vi "Match_Gauge Block.vi"(4 "Data in":string[][](array[string]), 5 "Calibration Default":string[][](array[string]), 6 "세부분류코드":string, 7 "Cal STD":string[][](array[string]), 8 "에러 입력":errorcluster caption="에러 입력(에러 없음)", 11 "Func_ext in":string) -> (0 "에러 출력":errorcluster, 1 "Data Out 2":string[](array[string]), 2 "Data Out":string[][](array[string]), 3 "CalSTD":string[][](array[string]))   [LabVIEW 2020]
uses:
  Controls/Cmd_File path.ctl
  Controls/Cmd_File Type.ctl
  Controls/Cmd_Var Data IO.ctl
  <vilib>/Utility/file.llb/Read Delimited Spreadsheet (string).vi
  Public/Polymorph/Data Class_2D Str.vi
  Public/Polymorph/Array Dedup_2D Str.vi
  Variables/Global_Cal Info.vi
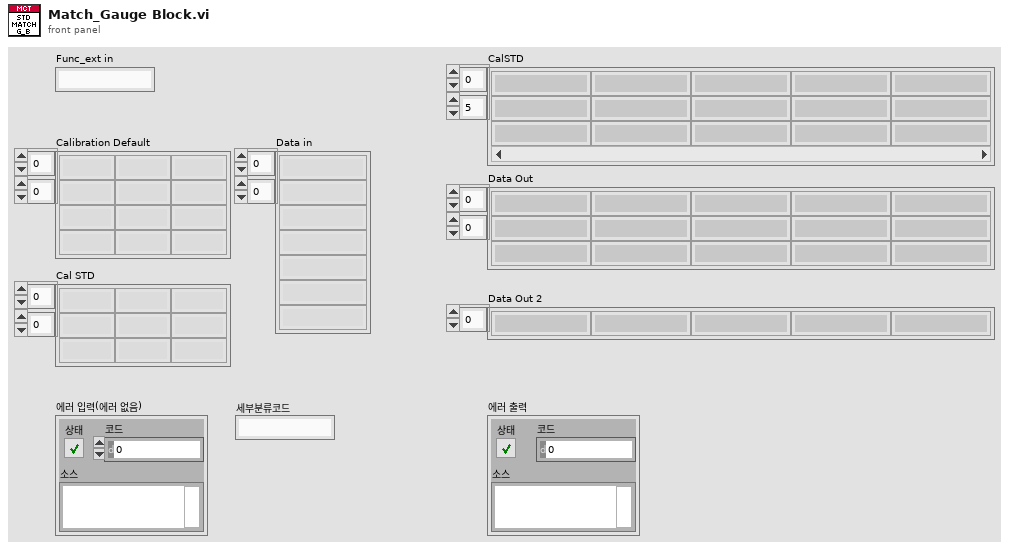
[diagram p1: front panel]
types:
  T1 = typedef "Cmd_File Type.ctl" = enum16{"엑셀", "엑셀(2003)", "텍스트", "설정", "2진", "VI", "CSV", "LOG", "폴더"}
  T2 = typedef "Cmd_File path.ctl" = enum16{"에러로그", "데이터파일경로", "성적서원본", "지난성적서", "Data Files", "경로생성", "Updater", "Template", "설정파일경로", "FTP Upload", "Update 경로", "어플리케이션"}
  T3 = typedef "Cmd_Var Data IO.ctl" = enum16{"Condition", "Condition Default", "Condition_Temp", "Resolution", "Resolution Default", "Resolution Old", "Spec", "Spec Default", "Spec Old", "Spec Temp", "Result", "Result2", "Result3", "Result_Temp", "Result_ADJ", "Result_ADJ2", "STD1", "STD2", "STD3", "STD4", "STD5", "STD Temp", "CMC", "CMC Default"}
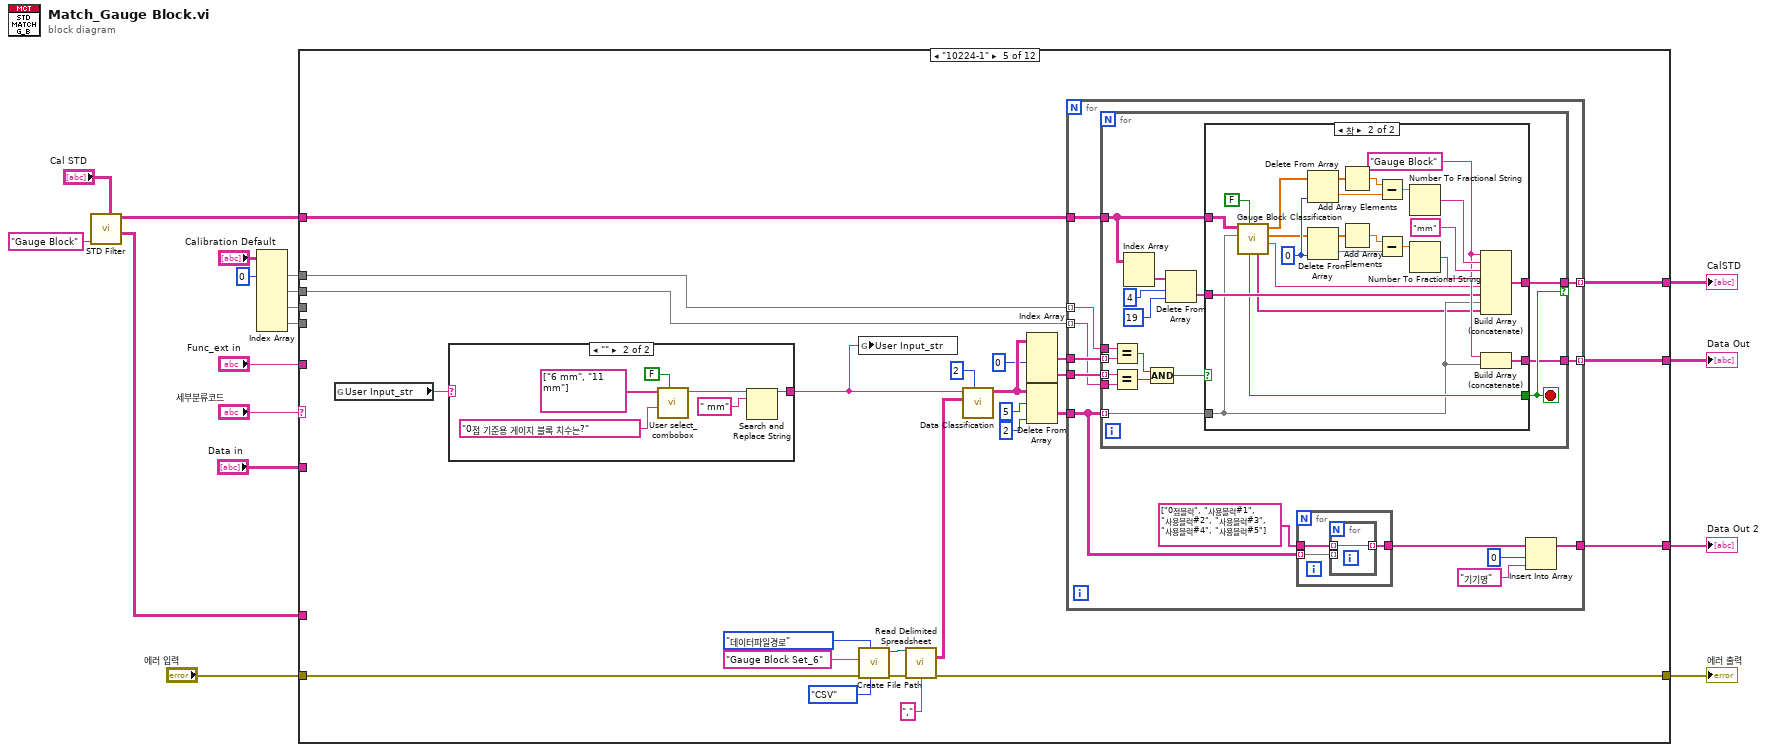
[diagram p0: block diagram]
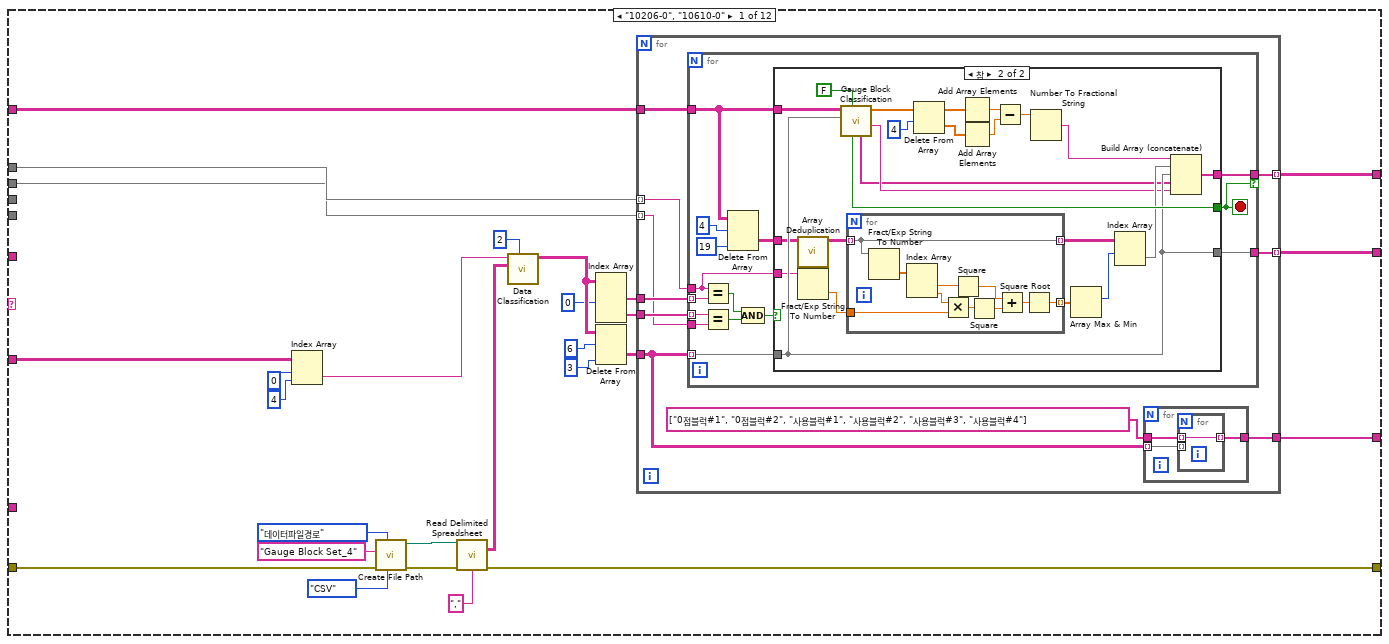
[diagram p2: hidden frame]
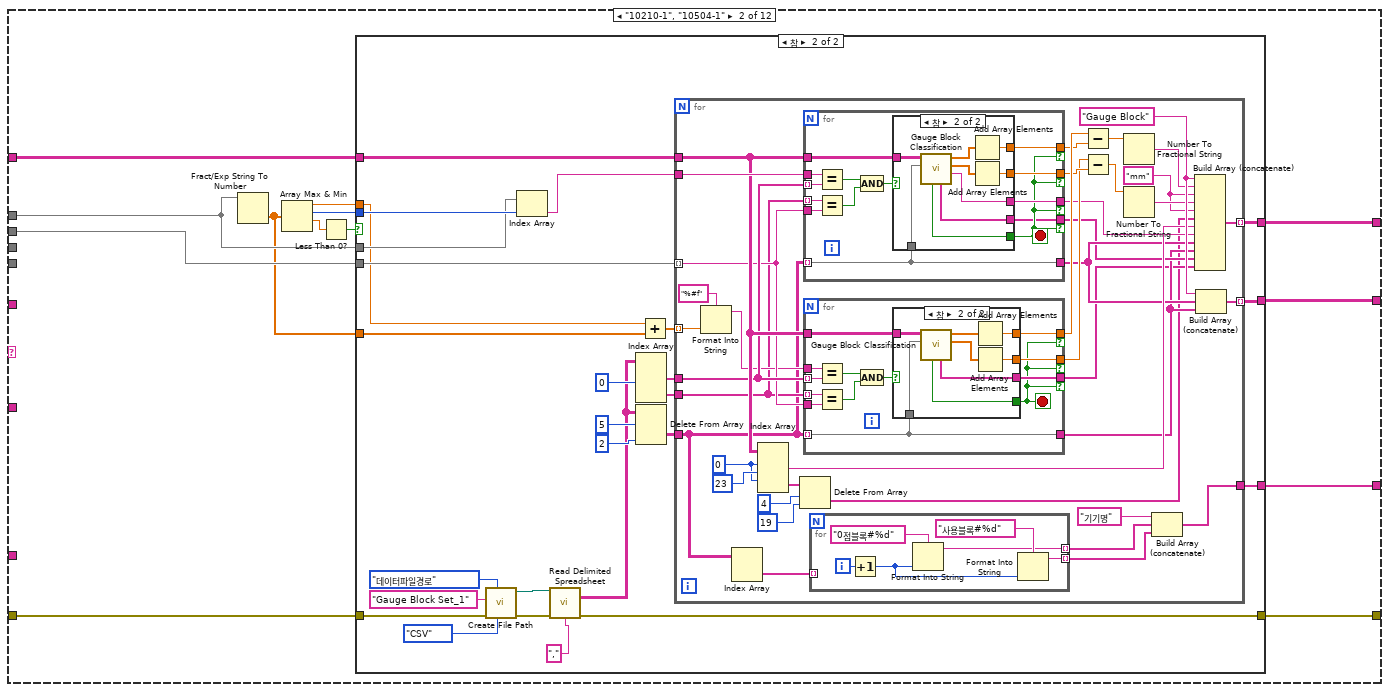
[diagram p4: hidden frame]
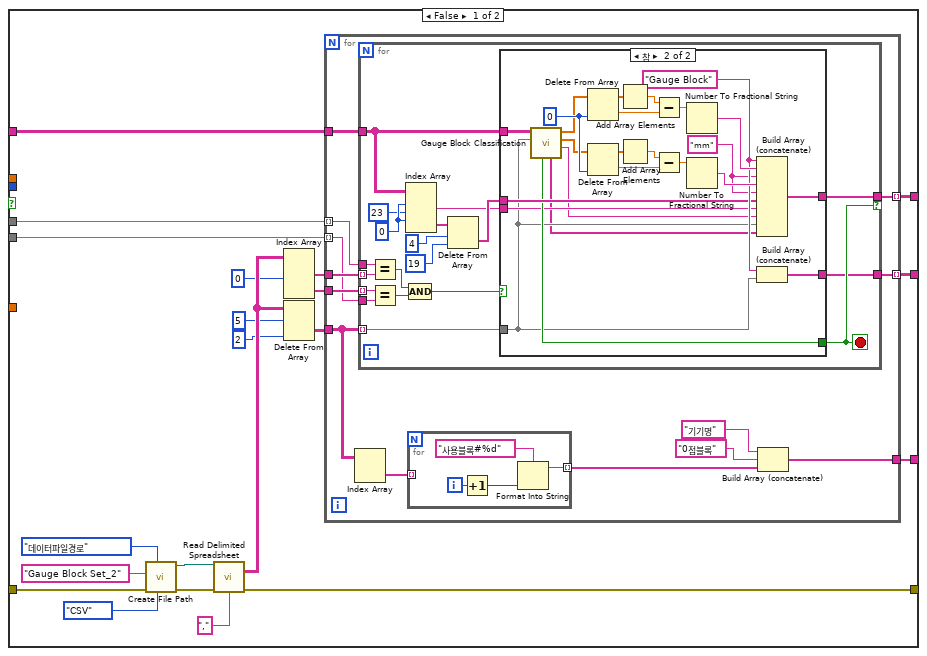
[diagram p5: hidden frame]
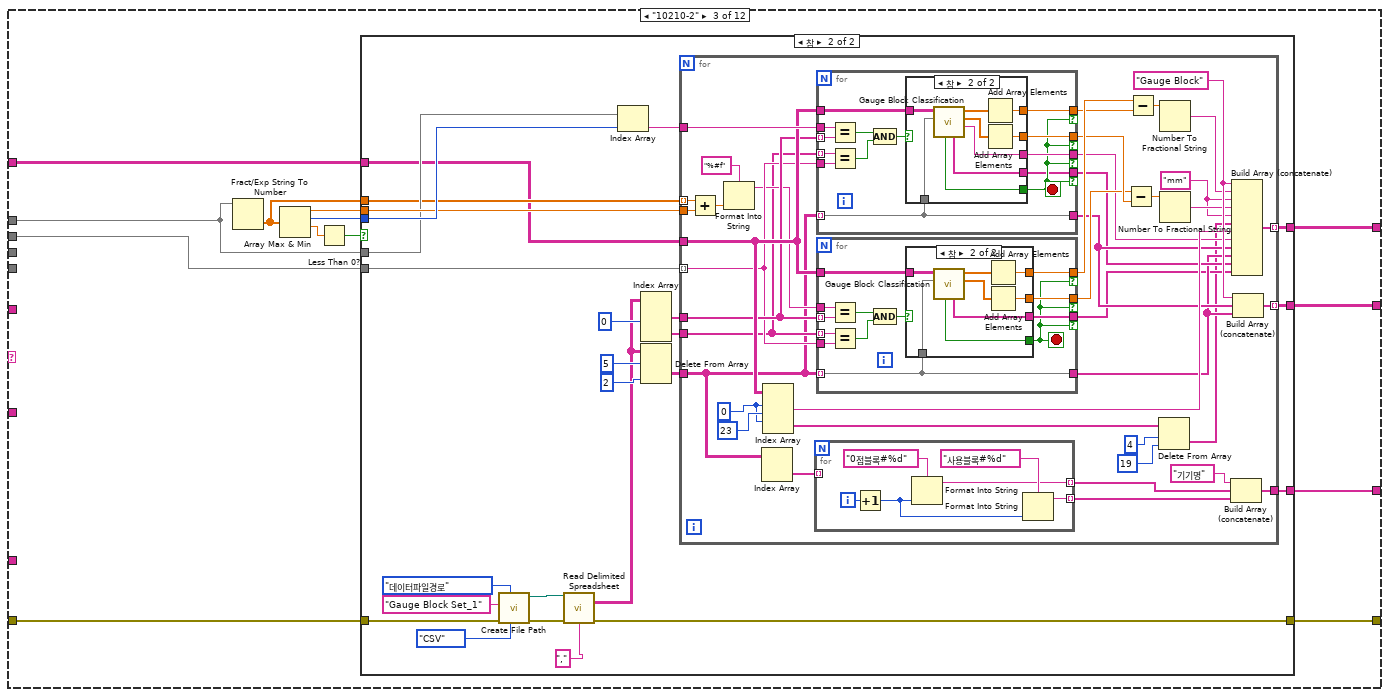
[diagram p9: hidden frame]
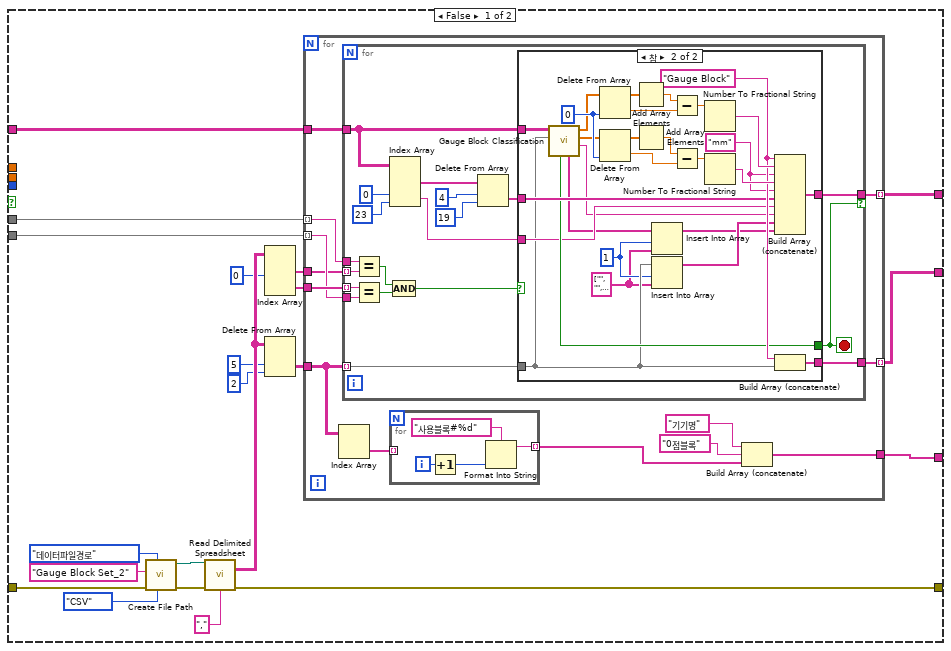
[diagram p10: hidden frame]
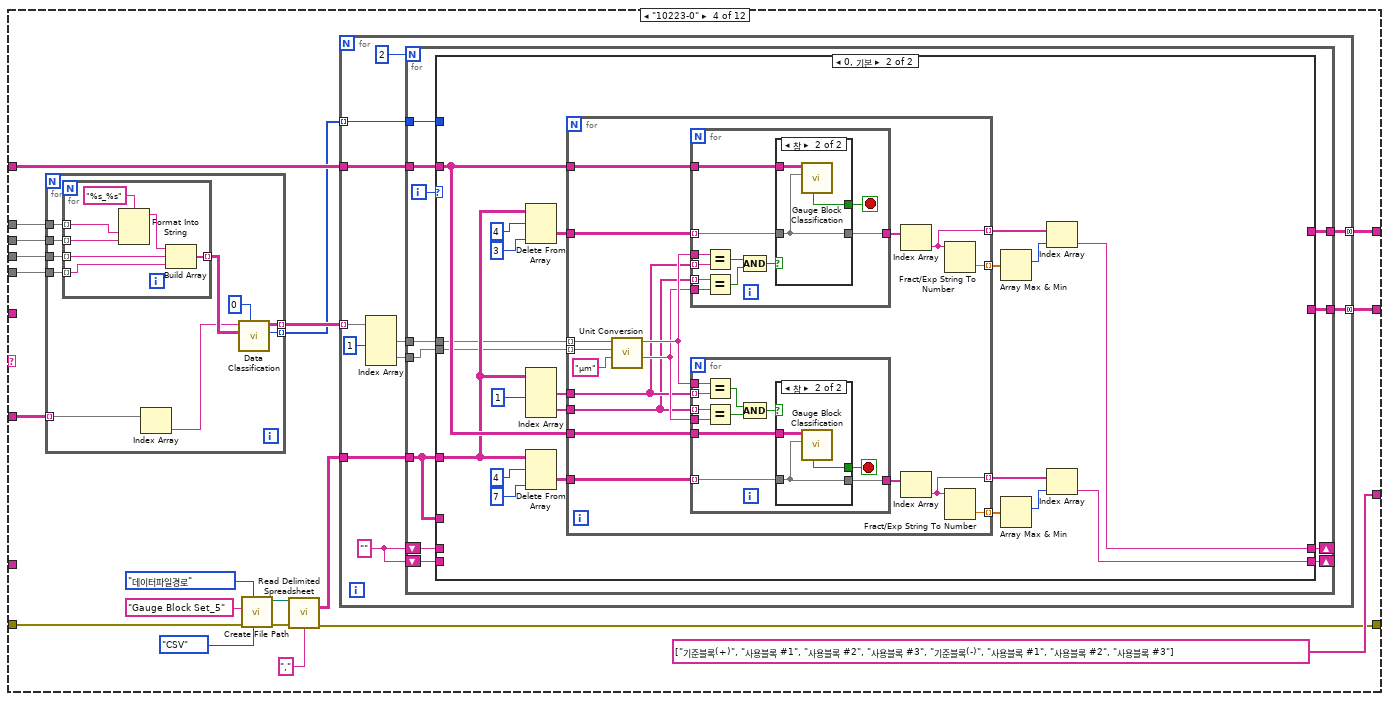
[diagram p14: hidden frame]
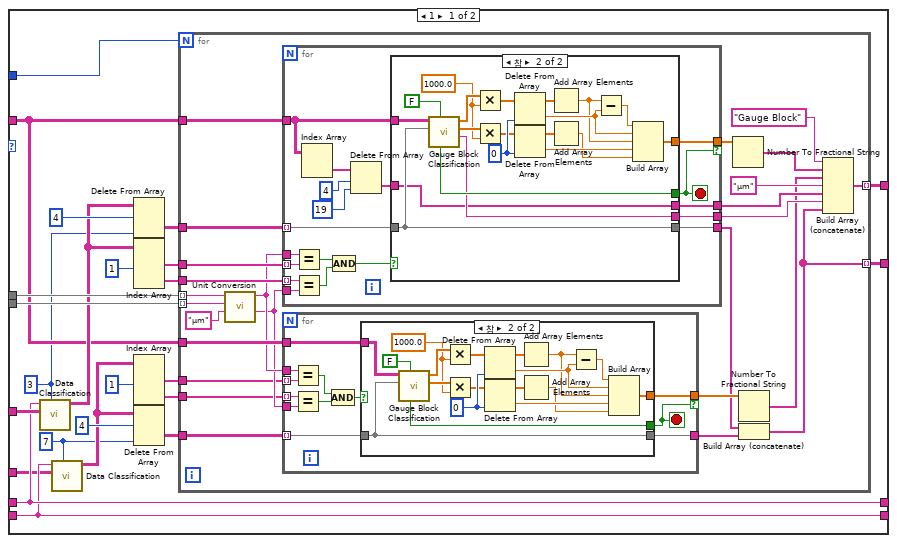
[diagram p15: hidden frame]
diagram:
  n1 = call "STD Filter.vi"("Cal STD in"="Cal STD", "문자열(option, STD)"="Gauge Block" ("검색 문자열")) -> ("Cal STD out"=w6:string[][], "DATA 출력"=w7:string[][])  [unwired: 5 in, 3 out]
  n2 = Index Array(array="Calibration Default", index (col) #1=0 ("비활성화된 인덱스 (열)")) -> (element #1=w10:string[], element #2=w9:string[], element #3=w2:string[], element #4=w1:string[])  [unwired: 7 in]
  n3 = case shown="\"10224-1\"" "세부분류코드" {
    tunnel: w10 -> [w28 w111 w326 w532 w782 w882 _ w1052 w1142 w1266 w1347 w1436]
    tunnel: w9 -> [w27 w112 w328 w531 w781 w881 w951 w1051 w1141 w1265 w1346 w1435]
    tunnel: w6 -> [_ _ _ _ _ w866 w957 _ _ w1250 w1331 w1420]
    tunnel: [w21 w120 w317 w548 w780 w880 w971 w1050 w1140 w1264 w1345 w1434] -> w13
    tunnel: [w20 w119 w318 w547 w779 w879 w970 w1049 w1139 w1263 w1344 w1433] -> w14
    tunnel: [w22 w116 w320 w535 w773 w861 w952 w1039 w1129 w1245 w1326 w1415] -> w16
    tunnel: "에러 입력" -> [w24 w118 w321 w537 w772 w864 w955 w1048 w1138 w1248 w1329 w1418]
    tunnel: [w19 w117 w319 string[] ["기준블록(+)", "사용블록 #1", "사용블록 #2", "사용블록 #3", "기준블록(-)", "사용블록 #1", "사용블록 #2", "사용블록 #3"] w778 w874 w965 w1043 w1133 w1258 w1339 w1428] -> w15
    tunnel: "Func_ext in" -> [_ _ _ _ _ w868 w959 _ _ w1252 w1333 w1422]
    tunnel: w7 -> [w26 w108 w316 w545 w775 w863 w954 w1041 w1131 w1247 w1328 w1417]
    tunnel: "Data in" -> [w25 _ _ w533 _ _ _ _ _ _ _ _]
    tunnel: w2 -> [_ _ _ w530 _ _ w950 _ _ _ _ _]
    tunnel: w1 -> [_ _ _ w529 _ _ _ _ _ _ _ _]
    frame "10206-0", "10610-0" {
      n4 = Index Array(array=w25, index (row)=0 ("인덱스 (행)"), index (col)=4 ("비활성화된 인덱스 (열)")) -> (element=w44:string)
      n5 = call "Create File Path.vi"("파일타입"=Cmd_File_Type."CSV", "항목"=Cmd_File_path."데이터파일경로", "에러 입력"=w24, "문자열 in"="Gauge Block Set_4" ("delimiter (\\t)")) -> ("error out"=w23:errorcluster, "파일경로"=w38:path)  [unwired: 4 in, 2 out]
      n6 = call-poly <vilib>:"Read Delimited Spreadsheet.vi"("file path (dialog if empty)"=w38, "error in (no error)"=w23, "delimiter (\\t)"="," ("delimiter (\\t)")) -> ("all rows"=w45:string[][], "error out"=w22:errorcluster)  [unwired: 7 in, 4 out]
      n7 = call-poly "Data Classification.vi"("인덱스"=2, "DATA 입력"=w45, "검색 문자열"=w44) -> ("DATA 출력"=w41:string[][])  [unwired: 4 in, 4 out]
      n8 = Index Array(array=w41, index (col) #1=0 ("비활성화된 인덱스 (열)")) -> (element #1=w30:string[], element #2=w29:string[])  [unwired: 3 in]
      n9 = Delete From Array(array=w41, length=6 ("길이"), index (col)=3 ("비활성화된 인덱스 (열)")) -> (deleted portion=w32:string[][])  [unwired: 1 in, 1 out]
      n10 = for {
        tunnel: w32 -> [w47]
        tunnel: w26 -> [w55]
        tunnel: w28 -> [w54] mode=indexing
        tunnel: w30 -> [w53]
        tunnel: w29 -> [w52]
        tunnel: w27 -> [w51] mode=indexing
        tunnel: [w50] -> w21 mode=indexing
        tunnel: [w49] -> w20 mode=indexing
        tunnel: [w46] -> w19
        n11 = for {
          tunnel: w54 -> [w56]
          tunnel: w51 -> [w70]
          tunnel: w47 -> [w67] mode=indexing
          tunnel: w55 -> [w60]
          tunnel: [w65] -> w50 if=w64
          tunnel: [w63] -> w49
          tunnel: w53 -> [w62] mode=indexing
          tunnel: w52 -> [w61] mode=indexing
          stop <- w64 stop-if-true
          n12 = Equal?(x=w56, y=w62) -> (x = y?=w68:bool)
          n13 = Equal?(x=w61, y=w70) -> (x = y?=w69:bool)
          n14 = Delete From Array(array=w60, length=4 ("길이"), index (col)=19 ("비활성화된 인덱스 (열)")) -> (deleted portion=w57:string[][])  [unwired: 1 in, 1 out]
          n15 = Compound Arithmetic op=AND(w68, w69) -> (w66:bool)
          n16 = case shown="참" w66 {
            tunnel: w67 -> [_ w87]
            tunnel: [_ w91] -> w64
            tunnel: w60 -> [_ w93]
            tunnel: [_ w92] -> w65
            tunnel: [_ w87] -> w63
            tunnel: w57 -> [_ w83]
            tunnel: w56 -> [_ w82]
            frame False {
            }
            frame True {
              n17 = call-poly "Array Deduplication.vi"("배열 in"=w83) -> ("배열 out"=w80:string[][])  [unwired: 9 in, 1 out]
              n18 = Fract/Exp String To Number(string=w82) -> (number=w81:dbl)  [unwired: 3 in, 1 out]
              n19 = call "Gauge Block Classification.vi"("블록삭제?(T)"=FALSE, "블록리스트"=w87, "게이지 블록 교정data"=w93) -> ("열팽창계수"=w73:string, "블록치수"=w88:dbl[], "교정값(문자)"=w72:string[], "stop?"=w91:bool)  [unwired: 3 in, 2 out]
              n20 = for {
                tunnel: w80 -> [w94] mode=indexing
                tunnel: w81 -> [w102]
                tunnel: [w95] -> w79 mode=indexing
                tunnel: [w94] -> w78 mode=indexing
                n21 = Fract/Exp String To Number(string=w94) -> (number=w103:dbl[])  [unwired: 3 in, 1 out]
                n22 = Index Array(array=w103) -> (element #1=w100:dbl, element #2=w101:dbl)  [unwired: 2 in]
                n23 = Multiply(x=w101, y=w102) -> (x*y=w99:dbl)
                n24 = Square(x=w100) -> (x^2=w98:dbl)
                n25 = Square(x=w99) -> (x^2=w97:dbl)
                n26 = Add(x=w98, y=w97) -> (x+y=w96:dbl)
                n27 = Square Root(x=w96) -> (sqrt(x)=w95:dbl)
              }
              n28 = Delete From Array(array=w88, length=4 ("길이")) -> (deleted portion=w90:dbl[], array with subset deleted=w75:dbl[])  [unwired: 1 in]
              n29 = Add Array Elements(numeric array=w75) -> (sum=w74:dbl)
              n30 = Add Array Elements(numeric array=w90) -> (sum=w84:dbl)
              n31 = Subtract(x=w74, y=w84) -> (x-y=w85:dbl)
              n32 = Number To Fractional String(number=w85) -> (F-format string=w89:string)  [unwired: 3 in]
              n33 = Array Max & Min(array=w79) -> (max index (indices)=w77:i32)  [unwired: 3 out]
              n34 = Index Array(array=w78, index (row)=w77) -> (element=w76:string[])  [unwired: 1 in]
              n35 = Build Array (concatenate)(w89, w76, w87, w72, w73) -> (w92:string[])
            }
          }
        }
        n36 = for {
          tunnel: w47 -> [w105] mode=indexing
          tunnel: string[] ["0점블럭#1", "0점블럭#2", "사용블럭#1", "사용블럭#2", "사용블럭#3", "사용블럭#4"] -> [w106]
          tunnel: [w104] -> w46
          n37 = for {
            tunnel: w106 -> [w107] mode=indexing
            tunnel: w105 -> [_] mode=indexing
            tunnel: [w107] -> w104 mode=indexing
          }
        }
      }
    }
    frame "10210-1", "10504-1" {
      n38 = Fract/Exp String To Number(string=w111) -> (number=w110:dbl[])  [unwired: 3 in, 1 out]
      n39 = Array Max & Min(array=w110) -> (max value=w113:dbl, max index (indices)=w114:i32, min value=w115:dbl)  [unwired: 1 out]
      n40 = Less Than 0?(x=w115) -> (x < 0?=w109:bool)
      n41 = case shown="참" w109 {
        tunnel: w108 -> [w129 w227]
        tunnel: [w125 w219] -> w120
        tunnel: [w124 w218] -> w119
        tunnel: w118 -> [w126 w217]
        tunnel: [w123 w212] -> w117
        tunnel: [w121 w202] -> w116
        tunnel: w114 -> [_ w209]
        tunnel: w113 -> [_ w206]
        tunnel: w112 -> [w128 w208]
        tunnel: w111 -> [w127 w207]
        tunnel: w110 -> [_ w205]
        frame False {
          n42 = call "Create File Path.vi"("파일타입"=Cmd_File_Type."CSV", "항목"=Cmd_File_path."데이터파일경로", "에러 입력"=w126, "문자열 in"="Gauge Block Set_2" ("delimiter (\\t)")) -> ("error out"=w122:errorcluster, "파일경로"=w140:path)  [unwired: 4 in, 2 out]
          n43 = call-poly <vilib>:"Read Delimited Spreadsheet.vi"("file path (dialog if empty)"=w140, "error in (no error)"=w122, "delimiter (\\t)"="," ("delimiter (\\t)")) -> ("all rows"=w141:string[][], "error out"=w121:errorcluster)  [unwired: 7 in, 4 out]
          n44 = Index Array(array=w141, index (col) #1=0 ("비활성화된 인덱스 (열)")) -> (element #1=w138:string[], element #2=w137:string[])  [unwired: 3 in]
          n45 = Delete From Array(array=w141, length=5 ("길이"), index (col)=2 ("비활성화된 인덱스 (열)")) -> (deleted portion=w139:string[][])  [unwired: 1 in, 1 out]
          n46 = for {
            tunnel: w139 -> [w144]
            tunnel: w129 -> [w154]
            tunnel: w127 -> [w153] mode=indexing
            tunnel: w138 -> [w152]
            tunnel: w137 -> [w151]
            tunnel: w128 -> [w150] mode=indexing
            tunnel: [w149] -> w125 mode=indexing
            tunnel: [w148] -> w124 mode=indexing
            tunnel: [w145] -> w123
            n47 = Index Array(array=w144) -> (element=w143:string[])  [unwired: 2 in]
            n48 = for {
              tunnel: w153 -> [w177]
              tunnel: w150 -> [w176]
              tunnel: w144 -> [w173] mode=indexing
              tunnel: w154 -> [w163]
              tunnel: [w171] -> w149 if=w170
              tunnel: [w169] -> w148
              tunnel: w152 -> [w168] mode=indexing
              tunnel: w151 -> [w167] mode=indexing
              stop <- w170 stop-if-true
              w161 = 0 ("인덱스 (행)")
              n49 = Equal?(x=w177, y=w168) -> (x = y?=w174:bool)
              n50 = Equal?(x=w167, y=w176) -> (x = y?=w175:bool)
              n51 = Index Array(array=w163, index (row) #1=w161, index (col) #1=23 ("비활성화된 인덱스 (열)"), index (row) #2=w161) -> (element #1=w159:string, element #2=w165:string[])  [unwired: 1 in]
              n52 = Compound Arithmetic op=AND(w174, w175) -> (w172:bool)
              n53 = Delete From Array(array=w165, length=4 ("길이"), index=19 ("비활성화된 인덱스 (열)")) -> (deleted portion=w162:string[])  [unwired: 1 out]
              n54 = case shown="참" w172 {
                tunnel: w173 -> [_ w179]
                tunnel: [_ w184] -> w170
                tunnel: w163 -> [_ w183]
                tunnel: [_ w201] -> w171
                tunnel: [_ w197] -> w169
                tunnel: w162 -> [_ w187]
                tunnel: w159 -> [_ w182]
                frame False {
                }
                frame True {
                  w190 = 0 ("인덱스")
                  w180 = "mm" ("환산단위")
                  w198 = "Gauge Block" ("검색 문자열")
                  n55 = call "Gauge Block Classification.vi"("블록리스트"=w179, "게이지 블록 교정data"=w183) -> ("열팽창계수"=w181:string, "교정값(값)"=w185:dbl[], "블록치수"=w186:dbl[], "교정값(문자)"=w178:string[], "stop?"=w184:bool)  [unwired: 4 in, 1 out]
                  n56 = Delete From Array(array=w186, index=w190) -> (deleted portion=w196:dbl, array with subset deleted=w192:dbl[])  [unwired: 1 in]
                  n57 = Delete From Array(array=w185, index=w190) -> (deleted portion=w194:dbl, array with subset deleted=w191:dbl[])  [unwired: 1 in]
                  n58 = Add Array Elements(numeric array=w192) -> (sum=w195:dbl)
                  n59 = Add Array Elements(numeric array=w191) -> (sum=w193:dbl)
                  n60 = Subtract(x=w195, y=w196) -> (x-y=w189:dbl)
                  n61 = Subtract(x=w193, y=w194) -> (x-y=w188:dbl)
                  n62 = Number To Fractional String(number=w189) -> (F-format string=w199:string)  [unwired: 3 in]
                  n63 = Number To Fractional String(number=w188) -> (F-format string=w200:string)  [unwired: 3 in]
                  n64 = Build Array (concatenate)(w198, w199, w180, w200, w180, w187, w182, w181, w179, w178) -> (w201:string[])
                  n65 = Build Array (concatenate)(w198, w179) -> (w197:string[])
                }
              }
            }
            n66 = for {
              tunnel: [w156] -> w147 mode=indexing
              tunnel: w143 -> [_] mode=indexing
              i -> [w157]
              n67 = Increment(x=w157) -> (x+1=w155:i32)
              n68 = Format Into String(format string="사용블록#%d" ("포맷 문자열"), w155) -> (resulting string=w156:string)  [unwired: 2 in, 1 out]
            }
            n69 = Build Array (concatenate)("기기명", "0점블록" ("포맷 문자열"), w147) -> (w145:string[])
          }
        }
        frame True {
          n70 = call "Create File Path.vi"("파일타입"=Cmd_File_Type."CSV", "항목"=Cmd_File_path."데이터파일경로", "에러 입력"=w217, "문자열 in"="Gauge Block Set_1" ("delimiter (\\t)")) -> ("error out"=w203:errorcluster, "파일경로"=w214:path)  [unwired: 4 in, 2 out]
          n71 = Index Array(array=w207, index=w209) -> (element=w210:string)
          n72 = call-poly <vilib>:"Read Delimited Spreadsheet.vi"("file path (dialog if empty)"=w214, "error in (no error)"=w203, "delimiter (\\t)"="," ("delimiter (\\t)")) -> ("all rows"=w211:string[][], "error out"=w202:errorcluster)  [unwired: 7 in, 4 out]
          n73 = Index Array(array=w211, index (col) #1=0 ("비활성화된 인덱스 (열)")) -> (element #1=w225:string[], element #2=w226:string[])  [unwired: 3 in]
          n74 = Delete From Array(array=w211, length=5 ("길이"), index (col)=2 ("비활성화된 인덱스 (열)")) -> (deleted portion=w223:string[][])  [unwired: 1 in, 1 out]
          n75 = Add(x=w206, y=w205) -> (x+y=w204:dbl[])
          n76 = for {
            tunnel: w223 -> [w232]
            tunnel: w227 -> [w262]
            tunnel: w225 -> [w261]
            tunnel: w226 -> [w239]
            tunnel: w208 -> [w260] mode=indexing
            tunnel: [w265] -> w219 mode=indexing
            tunnel: [w264] -> w218 mode=indexing
            tunnel: [w235] -> w212
            tunnel: w210 -> [w263]
            tunnel: w204 -> [w229] mode=indexing
            w243 = 0 ("인덱스 (행)")
            w228 = "mm" ("환산단위")
            w257 = "Gauge Block" ("검색 문자열")
            n77 = Format Into String(format string="%#f" ("포맷 문자열"), w229) -> (resulting string=w258:string)  [unwired: 2 in, 1 out]
            n78 = Index Array(array=w232) -> (element=w231:string[])  [unwired: 2 in]
            n79 = Index Array(array=w262, index (row) #1=w243, index (col) #1=23 ("비활성화된 인덱스 (열)"), index (row) #2=w243) -> (element #1=w247:string, element #2=w242:string[])  [unwired: 1 in]
            n80 = Delete From Array(array=w242, length=4 ("길이"), index=19 ("비활성화된 인덱스 (열)")) -> (deleted portion=w230:string[])  [unwired: 1 out]
            n81 = for {
              tunnel: w263 -> [w306]
              tunnel: w260 -> [w305]
              tunnel: w232 -> [w296] mode=indexing
              tunnel: w262 -> [w299]
              tunnel: [w293] -> w244 if=w294
              tunnel: [w296] -> w246
              tunnel: w261 -> [w301] mode=indexing
              tunnel: w239 -> [w300] mode=indexing
              tunnel: [w298] -> w252 if=w294
              tunnel: [w297] -> w253 if=w294
              tunnel: [w295] -> w245 if=w294
              stop <- w294 stop-if-true
              n82 = Equal?(x=w306, y=w301) -> (x = y?=w303:bool)
              n83 = Equal?(x=w300, y=w305) -> (x = y?=w304:bool)
              n84 = Compound Arithmetic op=AND(w303, w304) -> (w302:bool)
              n85 = case shown="참" w302 {
                tunnel: w296 -> [_ w312]
                tunnel: [_ w315] -> w294
                tunnel: w299 -> [_ w313]
                tunnel: [_ w311] -> w298
                tunnel: [_ w309] -> w297
                tunnel: [_ w308] -> w295
                tunnel: [_ w307] -> w293
                frame False {
                }
                frame True {
                  n86 = call "Gauge Block Classification.vi"("블록리스트"=w312, "게이지 블록 교정data"=w313) -> ("열팽창계수"=w308:string, "교정값(값)"=w314:dbl[], "블록치수"=w310:dbl[], "교정값(문자)"=w307:string[], "stop?"=w315:bool)  [unwired: 4 in, 1 out]
                  n87 = Add Array Elements(numeric array=w310) -> (sum=w309:dbl)
                  n88 = Add Array Elements(numeric array=w314) -> (sum=w311:dbl)
                }
              }
            }
            n89 = for {
              tunnel: w258 -> [w284]
              tunnel: w260 -> [w283]
              tunnel: w232 -> [w272] mode=indexing
              tunnel: w262 -> [w276]
              tunnel: [w279] -> w233 if=w273
              tunnel: [w272] -> w234
              tunnel: w261 -> [w278] mode=indexing
              tunnel: w239 -> [w277] mode=indexing
              tunnel: [w275] -> w256 if=w273
              tunnel: [w274] -> w251 if=w273
              stop <- w273 stop-if-true
              n90 = Equal?(x=w284, y=w278) -> (x = y?=w281:bool)
              n91 = Equal?(x=w277, y=w283) -> (x = y?=w282:bool)
              n92 = Compound Arithmetic op=AND(w281, w282) -> (w280:bool)
              n93 = case shown="참" w280 {
                tunnel: w272 -> [_ w288]
                tunnel: [_ w292] -> w273
                tunnel: w276 -> [_ w289]
                tunnel: [_ w285] -> w279
                tunnel: [_ w287] -> w275
                tunnel: [_ w286] -> w274
                frame False {
                }
                frame True {
                  n94 = call "Gauge Block Classification.vi"("블록리스트"=w288, "게이지 블록 교정data"=w289) -> ("교정값(값)"=w290:dbl[], "블록치수"=w291:dbl[], "교정값(문자)"=w285:string[], "stop?"=w292:bool)  [unwired: 4 in, 2 out]
                  n95 = Add Array Elements(numeric array=w291) -> (sum=w287:dbl)
                  n96 = Add Array Elements(numeric array=w290) -> (sum=w286:dbl)
                }
              }
            }
            n97 = for {
              tunnel: [w268] -> w238 mode=indexing
              tunnel: [w267] -> w237 mode=indexing
              tunnel: w231 -> [_] mode=indexing
              i -> [w269]
              n98 = Increment(x=w269) -> (x+1=w266:i32)
              n99 = Format Into String(format string="0점블록#%d" ("포맷 문자열"), w266) -> (resulting string=w268:string)  [unwired: 2 in, 1 out]
              n100 = Format Into String(format string="사용블록#%d" ("포맷 문자열"), w266) -> (resulting string=w267:string)  [unwired: 2 in, 1 out]
            }
            n101 = Subtract(x=w256, y=w253) -> (x-y=w255:dbl)
            n102 = Subtract(x=w251, y=w252) -> (x-y=w250:dbl)
            n103 = Number To Fractional String(number=w255) -> (F-format string=w254:string)  [unwired: 3 in]
            n104 = Number To Fractional String(number=w250) -> (F-format string=w249:string)  [unwired: 3 in]
            n105 = Build Array (concatenate)("기기명", w238, w237) -> (w235:string[])
            n106 = Build Array (concatenate)(w257, w254, w228, w249, w228, w230, w247, w245, w246, w234, w244, w233) -> (w265:string[])
            n107 = Build Array (concatenate)(w257, w246, w234) -> (w264:string[])
          }
        }
      }
    }
    frame "10210-2" {
      n108 = Fract/Exp String To Number(string=w326) -> (number=w322:dbl[])  [unwired: 3 in, 1 out]
      n109 = Array Max & Min(array=w322) -> (max value=w325:dbl, max index (indices)=w324:i32, min value=w327:dbl)  [unwired: 1 out]
      n110 = Less Than 0?(x=w327) -> (x < 0?=w323:bool)
      n111 = case shown="참" w323 {
        tunnel: [w336 w431] -> w317
        tunnel: [w335 w430] -> w318
        tunnel: w321 -> [w337 w429]
        tunnel: [w334 w424] -> w319
        tunnel: [w329 w414] -> w320
        tunnel: w324 -> [_ w421]
        tunnel: w325 -> [_ w420]
        tunnel: w328 -> [w339 w419]
        tunnel: w326 -> [w338 w418]
        tunnel: w322 -> [_ w417]
        tunnel: w316 -> [w331 w416]
        frame False {
          n112 = call "Create File Path.vi"("파일타입"=Cmd_File_Type."CSV", "항목"=Cmd_File_path."데이터파일경로", "에러 입력"=w337, "문자열 in"="Gauge Block Set_2" ("delimiter (\\t)")) -> ("error out"=w330:errorcluster, "파일경로"=w348:path)  [unwired: 4 in, 2 out]
          n113 = call-poly <vilib>:"Read Delimited Spreadsheet.vi"("file path (dialog if empty)"=w348, "error in (no error)"=w330, "delimiter (\\t)"="," ("delimiter (\\t)")) -> ("all rows"=w349:string[][], "error out"=w329:errorcluster)  [unwired: 7 in, 4 out]
          n114 = Index Array(array=w349, index (col) #1=0 ("비활성화된 인덱스 (열)")) -> (element #1=w333:string[], element #2=w332:string[])  [unwired: 3 in]
          n115 = Delete From Array(array=w349, length=5 ("길이"), index (col)=2 ("비활성화된 인덱스 (열)")) -> (deleted portion=w347:string[][])  [unwired: 1 in, 1 out]
          n116 = for {
            tunnel: w347 -> [w354]
            tunnel: w331 -> [w362]
            tunnel: w338 -> [w350] mode=indexing
            tunnel: w333 -> [w351]
            tunnel: w332 -> [w361]
            tunnel: w339 -> [w360] mode=indexing
            tunnel: [w359] -> w336 mode=indexing
            tunnel: [w358] -> w335 mode=indexing
            tunnel: [w355] -> w334
            n117 = Index Array(array=w354) -> (element=w353:string[])  [unwired: 2 in]
            n118 = for {
              tunnel: w350 -> [w385]
              tunnel: w360 -> [w384]
              tunnel: w354 -> [w382] mode=indexing
              tunnel: w362 -> [w373]
              tunnel: [w380] -> w359 if=w368
              tunnel: [w379] -> w358
              tunnel: w351 -> [w378] mode=indexing
              tunnel: w361 -> [w377] mode=indexing
              stop <- w368 stop-if-true
              n119 = Equal?(x=w385, y=w378) -> (x = y?=w367:bool)
              n120 = Equal?(x=w377, y=w384) -> (x = y?=w383:bool)
              n121 = Index Array(array=w373, index (row) #2=0 ("인덱스 (행)"), index (col) #2=23 ("비활성화된 인덱스 (열)")) -> (element #1=w375:string[], element #2=w369:string)  [unwired: 2 in]
              n122 = Compound Arithmetic op=AND(w367, w383) -> (w381:bool)
              n123 = Delete From Array(array=w375, length=4 ("길이"), index=19 ("비활성화된 인덱스 (열)")) -> (deleted portion=w372:string[])  [unwired: 1 out]
              n124 = case shown="참" w381 {
                tunnel: w382 -> [_ w393]
                tunnel: [_ w396] -> w368
                tunnel: w373 -> [_ w395]
                tunnel: [_ w413] -> w380
                tunnel: [_ w409] -> w379
                tunnel: w372 -> [_ w399]
                tunnel: w369 -> [_ w394]
                frame False {
                }
                frame True {
                  w390 = 1 ("인덱스")
                  w389 = string[] ["", "", "", ""]
                  w402 = 0 ("인덱스")
                  w386 = "mm" ("환산단위")
                  w410 = "Gauge Block" ("검색 문자열")
                  n125 = call "Gauge Block Classification.vi"("블록리스트"=w393, "게이지 블록 교정data"=w395) -> ("열팽창계수"=w388:string, "교정값(값)"=w397:dbl[], "블록치수"=w398:dbl[], "교정값(문자)"=w387:string[], "stop?"=w396:bool)  [unwired: 4 in, 1 out]
                  n126 = Delete From Array(array=w398, index=w402) -> (deleted portion=w408:dbl, array with subset deleted=w404:dbl[])  [unwired: 1 in]
                  n127 = Delete From Array(array=w397, index=w402) -> (deleted portion=w406:dbl, array with subset deleted=w403:dbl[])  [unwired: 1 in]
                  n128 = Add Array Elements(numeric array=w404) -> (sum=w407:dbl)
                  n129 = Add Array Elements(numeric array=w403) -> (sum=w405:dbl)
                  n130 = Insert Into Array(array=w387, index=w390, new element=w389) -> (w391:string[])
                  n131 = Insert Into Array(array=w393, index=w390, new element=w389) -> (w392:string[])
                  n132 = Subtract(x=w407, y=w408) -> (x-y=w401:dbl)
                  n133 = Subtract(x=w405, y=w406) -> (x-y=w400:dbl)
                  n134 = Number To Fractional String(number=w401) -> (F-format string=w411:string)  [unwired: 3 in]
                  n135 = Number To Fractional String(number=w400) -> (F-format string=w412:string)  [unwired: 3 in]
                  n136 = Build Array (concatenate)(w410, w411, w386, w412, w386, w399, w394, w388, w392, w391) -> (w413:string[])
                  n137 = Build Array (concatenate)(w410, w393) -> (w409:string[])
                }
              }
            }
            n138 = for {
              tunnel: [w364] -> w357 mode=indexing
              tunnel: w353 -> [_] mode=indexing
              i -> [w365]
              n139 = Increment(x=w365) -> (x+1=w363:i32)
              n140 = Format Into String(format string="사용블록#%d" ("포맷 문자열"), w363) -> (resulting string=w364:string)  [unwired: 2 in, 1 out]
            }
            n141 = Build Array (concatenate)("기기명", "0점블록" ("포맷 문자열"), w357) -> (w355:string[])
          }
        }
        frame True {
          n142 = call "Create File Path.vi"("파일타입"=Cmd_File_Type."CSV", "항목"=Cmd_File_path."데이터파일경로", "에러 입력"=w429, "문자열 in"="Gauge Block Set_1" ("delimiter (\\t)")) -> ("error out"=w415:errorcluster, "파일경로"=w426:path)  [unwired: 4 in, 2 out]
          n143 = call-poly <vilib>:"Read Delimited Spreadsheet.vi"("file path (dialog if empty)"=w426, "error in (no error)"=w415, "delimiter (\\t)"="," ("delimiter (\\t)")) -> ("all rows"=w423:string[][], "error out"=w414:errorcluster)  [unwired: 7 in, 4 out]
          n144 = Index Array(array=w418, index=w421) -> (element=w422:string)
          n145 = Index Array(array=w423, index (col) #1=0 ("비활성화된 인덱스 (열)")) -> (element #1=w437:string[], element #2=w438:string[])  [unwired: 3 in]
          n146 = Delete From Array(array=w423, length=5 ("길이"), index (col)=2 ("비활성화된 인덱스 (열)")) -> (deleted portion=w435:string[][])  [unwired: 1 in, 1 out]
          n147 = for {
            tunnel: w435 -> [w442]
            tunnel: w416 -> [w475]
            tunnel: w437 -> [w472]
            tunnel: w438 -> [w449]
            tunnel: w419 -> [w471] mode=indexing
            tunnel: [w478] -> w431 mode=indexing
            tunnel: [w477] -> w430 mode=indexing
            tunnel: [w445] -> w424
            tunnel: w422 -> [w476]
            tunnel: w420 -> [w474]
            tunnel: w417 -> [w473] mode=indexing
            w453 = 0 ("인덱스 (행)")
            w439 = "mm" ("환산단위")
            w467 = "Gauge Block" ("검색 문자열")
            n148 = Add(x=w473, y=w474) -> (x+y=w470:dbl)
            n149 = Format Into String(format string="%#f" ("포맷 문자열"), w470) -> (resulting string=w468:string)  [unwired: 2 in, 1 out]
            n150 = Index Array(array=w442) -> (element=w441:string[])  [unwired: 2 in]
            n151 = Index Array(array=w475, index (row) #1=w453, index (col) #1=23 ("비활성화된 인덱스 (열)"), index (row) #2=w453) -> (element #1=w457:string, element #2=w452:string[])  [unwired: 1 in]
            n152 = for {
              tunnel: [w481] -> w448 mode=indexing
              tunnel: [w480] -> w447 mode=indexing
              tunnel: w441 -> [_] mode=indexing
              i -> [w482]
              n153 = Increment(x=w482) -> (x+1=w479:i32)
              n154 = Format Into String(format string="0점블록#%d" ("포맷 문자열"), w479) -> (resulting string=w481:string)  [unwired: 2 in, 1 out]
              n155 = Format Into String(format string="사용블록#%d" ("포맷 문자열"), w479) -> (resulting string=w480:string)  [unwired: 2 in, 1 out]
            }
            n156 = for {
              tunnel: w476 -> [w519]
              tunnel: w471 -> [w518]
              tunnel: w442 -> [w509] mode=indexing
              tunnel: w475 -> [w512]
              tunnel: [w506] -> w454 if=w507
              tunnel: [w509] -> w456
              tunnel: w472 -> [w514] mode=indexing
              tunnel: w449 -> [w513] mode=indexing
              tunnel: [w511] -> w462 if=w507
              tunnel: [w510] -> w463 if=w507
              tunnel: [w508] -> w455 if=w507
              stop <- w507 stop-if-true
              n157 = Equal?(x=w519, y=w514) -> (x = y?=w516:bool)
              n158 = Equal?(x=w513, y=w518) -> (x = y?=w517:bool)
              n159 = Compound Arithmetic op=AND(w516, w517) -> (w515:bool)
              n160 = case shown="참" w515 {
                tunnel: w509 -> [_ w525]
                tunnel: [_ w528] -> w507
                tunnel: w512 -> [_ w526]
                tunnel: [_ w524] -> w511
                tunnel: [_ w522] -> w510
                tunnel: [_ w521] -> w508
                tunnel: [_ w520] -> w506
                frame False {
                }
                frame True {
                  n161 = call "Gauge Block Classification.vi"("블록리스트"=w525, "게이지 블록 교정data"=w526) -> ("열팽창계수"=w521:string, "교정값(값)"=w527:dbl[], "블록치수"=w523:dbl[], "교정값(문자)"=w520:string[], "stop?"=w528:bool)  [unwired: 4 in, 1 out]
                  n162 = Add Array Elements(numeric array=w523) -> (sum=w522:dbl)
                  n163 = Add Array Elements(numeric array=w527) -> (sum=w524:dbl)
                }
              }
            }
            n164 = for {
              tunnel: w468 -> [w497]
              tunnel: w471 -> [w496]
              tunnel: w442 -> [w485] mode=indexing
              tunnel: w475 -> [w489]
              tunnel: [w492] -> w443 if=w486
              tunnel: [w485] -> w444
              tunnel: w472 -> [w491] mode=indexing
              tunnel: w449 -> [w490] mode=indexing
              tunnel: [w488] -> w466 if=w486
              tunnel: [w487] -> w461 if=w486
              stop <- w486 stop-if-true
              n165 = Equal?(x=w497, y=w491) -> (x = y?=w494:bool)
              n166 = Equal?(x=w490, y=w496) -> (x = y?=w495:bool)
              n167 = Compound Arithmetic op=AND(w494, w495) -> (w493:bool)
              n168 = case shown="참" w493 {
                tunnel: w485 -> [_ w501]
                tunnel: [_ w505] -> w486
                tunnel: w489 -> [_ w502]
                tunnel: [_ w498] -> w492
                tunnel: [_ w500] -> w488
                tunnel: [_ w499] -> w487
                frame False {
                }
                frame True {
                  n169 = call "Gauge Block Classification.vi"("블록리스트"=w501, "게이지 블록 교정data"=w502) -> ("교정값(값)"=w503:dbl[], "블록치수"=w504:dbl[], "교정값(문자)"=w498:string[], "stop?"=w505:bool)  [unwired: 4 in, 2 out]
                  n170 = Add Array Elements(numeric array=w504) -> (sum=w500:dbl)
                  n171 = Add Array Elements(numeric array=w503) -> (sum=w499:dbl)
                }
              }
            }
            n172 = Subtract(x=w461, y=w462) -> (x-y=w460:dbl)
            n173 = Subtract(x=w466, y=w463) -> (x-y=w465:dbl)
            n174 = Delete From Array(array=w452, length=4 ("길이"), index=19 ("비활성화된 인덱스 (열)")) -> (deleted portion=w440:string[])  [unwired: 1 out]
            n175 = Number To Fractional String(number=w465) -> (F-format string=w464:string)  [unwired: 3 in]
            n176 = Number To Fractional String(number=w460) -> (F-format string=w459:string)  [unwired: 3 in]
            n177 = Build Array (concatenate)("기기명", w448, w447) -> (w445:string[])
            n178 = Build Array (concatenate)(w467, w464, w439, w459, w439, w440, w457, w455, w456, w444, w454, w443) -> (w478:string[])
            n179 = Build Array (concatenate)(w467, w456, w444) -> (w477:string[])
          }
        }
      }
    }
    frame "10223-0" {
      n180 = for {
        tunnel: w533 -> [w557] mode=indexing
        tunnel: [w554] -> w544 mode=indexing
        tunnel: [w553] -> w543 mode=indexing
        tunnel: w532 -> [w552]
        tunnel: w531 -> [w551]
        tunnel: w530 -> [w550]
        tunnel: w529 -> [w549]
        n181 = for {
          tunnel: [w563] -> w558 mode=indexing
          tunnel: w552 -> [w564] mode=indexing
          tunnel: w551 -> [w562] mode=indexing
          tunnel: w550 -> [w560] mode=indexing
          tunnel: w549 -> [w559] mode=indexing
          n182 = Format Into String(format string="%s_%s" ("포맷 문자열"), w564, w562) -> (resulting string=w561:string)  [unwired: 2 in, 1 out]
          n183 = Build Array(w561, w560, w559) -> (w563:string[])
        }
        n184 = Index Array(array=w557) -> (element=w556:string)  [unwired: 1 in]
        n185 = call-poly "Data Classification.vi"("인덱스"=0, "DATA 입력"=w558, "검색 문자열"=w556) -> ("행크기"=w553:i32, "DATA 출력"=w554:string[][])  [unwired: 4 in, 3 out]
      }
      n186 = call "Create File Path.vi"("파일타입"=Cmd_File_Type."CSV", "항목"=Cmd_File_path."데이터파일경로", "에러 입력"=w537, "문자열 in"="Gauge Block Set_5" ("delimiter (\\t)")) -> ("error out"=w536:errorcluster, "파일경로"=w541:path)  [unwired: 4 in, 2 out]
      n187 = call-poly <vilib>:"Read Delimited Spreadsheet.vi"("file path (dialog if empty)"=w541, "error in (no error)"=w536, "delimiter (\\t)"="," ("delimiter (\\t)")) -> ("all rows"=w534:string[][], "error out"=w535:errorcluster)  [unwired: 7 in, 4 out]
      n188 = for {
        tunnel: w534 -> [w574]
        tunnel: w545 -> [w573]
        tunnel: w544 -> [w571] mode=indexing
        tunnel: [w570] -> w547 mode=concatenating
        tunnel: [w568] -> w548 mode=concatenating
        tunnel: w543 -> [w567] mode=indexing
        w569 = "" ("String")
        n189 = Index Array(array=w571, index (col) #1=1 ("비활성화된 인덱스 (열)")) -> (element #1=w576:string[], element #2=w575:string[])  [unwired: 3 in]
        n190 = for {
          N: 2 -> [_]
          tunnel: w576 -> [w588]
          tunnel: w575 -> [w587]
          tunnel: [w579] -> w568
          tunnel: w574 -> [w580]
          tunnel: w573 -> [w586]
          shift-right: [w585] -> _
          shift-left: w569 -> [w584]
          tunnel: [w578] -> w570
          shift-right: [w581] -> _
          shift-left: w569 -> [w582]
          tunnel: w567 -> [w577]
          i -> [w583]
          n191 = case shown="0, 기본" w583 {
            tunnel: w588 -> [w607 w707]
            tunnel: w587 -> [w606 w706]
            tunnel: [w605 _] -> w579
            tunnel: [w604 _] -> w578
            tunnel: w586 -> [w600 w717]
            tunnel: [w601 w709] -> w585
            tunnel: w580 -> [w603 w708]
            tunnel: w584 -> [w601 _]
            tunnel: w582 -> [w599 _]
            tunnel: [w599 w710] -> w581
            tunnel: w580 -> [w598 _]
            tunnel: w577 -> [w589 _]
            frame 1 {
              w590 = 7 ("인덱스")
              w591 = 3 ("인덱스")
              n192 = call-poly "Data Classification.vi"("인덱스"=w591, "DATA 입력"=w603, "검색 문자열"=w601) -> ("DATA 출력"=w602:string[][])  [unwired: 4 in, 4 out]
              n193 = call-poly "Data Classification.vi"("인덱스"=w590, "DATA 입력"=w598, "검색 문자열"=w599) -> ("DATA 출력"=w593:string[][])  [unwired: 4 in, 4 out]
              n194 = Delete From Array(array=w602, length=4 ("길이"), index (col)=w591) -> (deleted portion=w609:string[][])  [unwired: 1 in, 1 out]
              n195 = Index Array(array=w602, index (col) #1=1 ("비활성화된 인덱스 (열)")) -> (element #1=w611:string[], element #2=w612:string[])  [unwired: 3 in]
              n196 = Index Array(array=w593, index (col) #1=1 ("비활성화된 인덱스 (열)")) -> (element #1=w596:string[], element #2=w595:string[])  [unwired: 3 in]
              n197 = Delete From Array(array=w593, length=4 ("길이"), index (col)=w590) -> (deleted portion=w592:string[][])  [unwired: 1 in, 1 out]
              n198 = for {
                N: w589 -> [_]
                tunnel: w609 -> [w634]
                tunnel: w600 -> [w637]
                tunnel: w607 -> [w633] mode=indexing
                tunnel: w611 -> [w636]
                tunnel: w612 -> [w635]
                tunnel: w606 -> [w632] mode=indexing
                tunnel: [w623] -> w605 mode=indexing
                tunnel: [w616] -> w604 mode=indexing
                tunnel: w600 -> [w630]
                tunnel: w596 -> [w627]
                tunnel: w595 -> [w626]
                tunnel: w592 -> [w625]
                n199 = call "Unit Conversion.vi"("환산단위"="μm", "입력단위"=w632, "입력값"=w633) -> ("환산단위"=w628:string, "환산값 (string)"=w629:string)  [unwired: 3 in, 4 out]
                n200 = for {
                  tunnel: w629 -> [w685]
                  tunnel: w628 -> [w684]
                  tunnel: w634 -> [w681] mode=indexing
                  tunnel: w637 -> [w675]
                  tunnel: [w679] -> w615 if=w678
                  tunnel: [w677] -> w618
                  tunnel: w636 -> [w674] mode=indexing
                  tunnel: w635 -> [w676] mode=indexing
                  tunnel: [w668] -> w620
                  tunnel: [w673] -> w619
                  stop <- w678 stop-if-true
                  n201 = Equal?(x=w685, y=w674) -> (x = y?=w682:bool)
                  n202 = Equal?(x=w676, y=w684) -> (x = y?=w683:bool)
                  n203 = Index Array(array=w675) -> (element=w672:string[])  [unwired: 2 in]
                  n204 = Compound Arithmetic op=AND(w682, w683) -> (w680:bool)
                  n205 = Delete From Array(array=w672, length=4 ("길이"), index=19 ("비활성화된 인덱스 (열)")) -> (deleted portion=w669:string[])  [unwired: 1 out]
                  n206 = case shown="참" w680 {
                    tunnel: w681 -> [_ w699]
                    tunnel: [_ w700] -> w678
                    tunnel: w675 -> [_ w696]
                    tunnel: [_ w705] -> w679
                    tunnel: [_ w699] -> w677
                    tunnel: [_ w697] -> w673
                    tunnel: w669 -> [_ w695]
                    tunnel: [_ w695] -> w668
                    frame False {
                    }
                    frame True {
                      w691 = 1000.0 ("y")
                      w703 = 0 ("인덱스")
                      n207 = call "Gauge Block Classification.vi"("블록삭제?(T)"=FALSE, "블록리스트"=w699, "게이지 블록 교정data"=w696) -> ("열팽창계수"=w697:string, "교정값(값)"=w701:dbl[], "블록치수"=w702:dbl[], "stop?"=w700:bool)  [unwired: 3 in, 2 out]
                      n208 = Multiply(x=w702, y=w691) -> (x*y=w693:dbl[])
                      n209 = Multiply(x=w701, y=w691) -> (x*y=w692:dbl[])
                      n210 = Delete From Array(array=w693, index=w703) -> (deleted portion=w689:dbl, array with subset deleted=w694:dbl[])  [unwired: 1 in]
                      n211 = Delete From Array(array=w692, index=w703) -> (deleted portion=w687:dbl, array with subset deleted=w704:dbl[])  [unwired: 1 in]
                      n212 = Add Array Elements(numeric array=w694) -> (sum=w688:dbl)
                      n213 = Add Array Elements(numeric array=w704) -> (sum=w686:dbl)
                      n214 = Subtract(x=w688, y=w689) -> (x-y=w690:dbl)
                      n215 = Build Array(w690, w689, w688, w687, w686) -> (w705:dbl[])
                    }
                  }
                }
                n216 = for {
                  tunnel: w629 -> [w649]
                  tunnel: w628 -> [w648]
                  tunnel: w625 -> [w641] mode=indexing
                  tunnel: w630 -> [w643]
                  tunnel: [w640] -> w622 if=w639
                  tunnel: [w638] -> w617
                  tunnel: w627 -> [w644] mode=indexing
                  tunnel: w626 -> [w645] mode=indexing
                  stop <- w639 stop-if-true
                  n217 = Equal?(x=w649, y=w644) -> (x = y?=w646:bool)
                  n218 = Equal?(x=w645, y=w648) -> (x = y?=w647:bool)
                  n219 = Compound Arithmetic op=AND(w646, w647) -> (w642:bool)
                  n220 = case shown="참" w642 {
                    tunnel: w641 -> [_ w655]
                    tunnel: [_ w662] -> w639
                    tunnel: w643 -> [_ w660]
                    tunnel: [_ w667] -> w640
                    tunnel: [_ w655] -> w638
                    frame False {
                    }
                    frame True {
                      w656 = 1000.0 ("y")
                      w665 = 0 ("인덱스")
                      n221 = call "Gauge Block Classification.vi"("블록삭제?(T)"=FALSE, "블록리스트"=w655, "게이지 블록 교정data"=w660) -> ("교정값(값)"=w663:dbl[], "블록치수"=w664:dbl[], "stop?"=w662:bool)  [unwired: 3 in, 3 out]
                      n222 = Multiply(x=w664, y=w656) -> (x*y=w658:dbl[])
                      n223 = Multiply(x=w663, y=w656) -> (x*y=w657:dbl[])
                      n224 = Delete From Array(array=w658, index=w665) -> (deleted portion=w653:dbl, array with subset deleted=w659:dbl[])  [unwired: 1 in]
                      n225 = Delete From Array(array=w657, index=w665) -> (deleted portion=w651:dbl, array with subset deleted=w666:dbl[])  [unwired: 1 in]
                      n226 = Add Array Elements(numeric array=w659) -> (sum=w652:dbl)
                      n227 = Add Array Elements(numeric array=w666) -> (sum=w650:dbl)
                      n228 = Subtract(x=w652, y=w653) -> (x-y=w654:dbl)
                      n229 = Build Array(w654, w653, w652, w651, w650) -> (w667:dbl[])
                    }
                  }
                }
                n230 = Number To Fractional String(number=w615) -> (F-format string=w614:string[])  [unwired: 3 in]
                n231 = Number To Fractional String(number=w622) -> (F-format string=w613:string[])  [unwired: 3 in]
                n232 = Build Array (concatenate)(w618, w617) -> (w616:string[])
                n233 = Build Array (concatenate)("Gauge Block", w614, w613, "μm" ("원소"), w620, w619, w616) -> (w623:string[])
              }
            }
            frame 0, Default {
              n234 = Delete From Array(array=w708, length=4 ("길이"), index (col)=3 ("비활성화된 인덱스 (열)")) -> (deleted portion=w723:string[][])  [unwired: 1 in, 1 out]
              n235 = Index Array(array=w708, index (col) #1=1 ("비활성화된 인덱스 (열)")) -> (element #1=w725:string[], element #2=w726:string[])  [unwired: 3 in]
              n236 = Delete From Array(array=w708, length=4 ("길이"), index (col)=7 ("비활성화된 인덱스 (열)")) -> (deleted portion=w714:string[][])  [unwired: 1 in, 1 out]
              n237 = for {
                tunnel: w723 -> [w727]
                tunnel: w717 -> [w743]
                tunnel: w707 -> [w742] mode=indexing
                tunnel: w725 -> [w733]
                tunnel: w726 -> [w732]
                tunnel: w706 -> [w741] mode=indexing
                tunnel: [w739] -> w720 mode=indexing
                tunnel: [w738] -> w719 mode=indexing
                tunnel: w717 -> [w734]
                tunnel: w714 -> [w731]
                tunnel: [w729] -> w712 mode=indexing
                tunnel: [w728] -> w711 mode=indexing
                n238 = call "Unit Conversion.vi"("환산단위"="μm", "입력단위"=w741, "입력값"=w742) -> ("환산단위"=w735:string, "환산값 (string)"=w736:string)  [unwired: 3 in, 4 out]
                n239 = for {
                  tunnel: w736 -> [w768]
                  tunnel: w735 -> [w767]
                  tunnel: w727 -> [w764] mode=indexing
                  tunnel: w743 -> [w759]
                  tunnel: [w761] -> w737
                  tunnel: w733 -> [w758] mode=indexing
                  tunnel: w732 -> [w760] mode=indexing
                  stop <- w762 stop-if-true
                  n240 = Equal?(x=w768, y=w758) -> (x = y?=w765:bool)
                  n241 = Equal?(x=w760, y=w767) -> (x = y?=w766:bool)
                  n242 = Compound Arithmetic op=AND(w765, w766) -> (w763:bool)
                  n243 = case shown="참" w763 {
                    tunnel: w764 -> [_ w769]
                    tunnel: [_ w771] -> w762
                    tunnel: w759 -> [_ w770]
                    tunnel: [_ w769] -> w761
                    frame False {
                    }
                    frame True {
                      n244 = call "Gauge Block Classification.vi"("블록리스트"=w769, "게이지 블록 교정data"=w770) -> ("stop?"=w771:bool)  [unwired: 4 in, 5 out]
                    }
                  }
                }
                n245 = for {
                  tunnel: w736 -> [w754]
                  tunnel: w735 -> [w753]
                  tunnel: w731 -> [w750] mode=indexing
                  tunnel: w734 -> [w745]
                  tunnel: [w747] -> w730
                  tunnel: w733 -> [w744] mode=indexing
                  tunnel: w732 -> [w746] mode=indexing
                  stop <- w748 stop-if-true
                  n246 = Equal?(x=w754, y=w744) -> (x = y?=w751:bool)
                  n247 = Equal?(x=w746, y=w753) -> (x = y?=w752:bool)
                  n248 = Compound Arithmetic op=AND(w751, w752) -> (w749:bool)
                  n249 = case shown="참" w749 {
                    tunnel: w750 -> [_ w755]
                    tunnel: [_ w757] -> w748
                    tunnel: w745 -> [_ w756]
                    tunnel: [_ w755] -> w747
                    frame False {
                    }
                    frame True {
                      n250 = call "Gauge Block Classification.vi"("블록리스트"=w755, "게이지 블록 교정data"=w756) -> ("stop?"=w757:bool)  [unwired: 4 in, 5 out]
                    }
                  }
                }
                n251 = Index Array(array=w737) -> (element=w738:string)  [unwired: 1 in]
                n252 = Index Array(array=w730) -> (element=w728:string)  [unwired: 1 in]
                n253 = Fract/Exp String To Number(string=w738) -> (number=w739:dbl)  [unwired: 3 in, 1 out]
                n254 = Fract/Exp String To Number(string=w728) -> (number=w729:dbl)  [unwired: 3 in, 1 out]
              }
              n255 = Array Max & Min(array=w720) -> (max index (indices)=w718:i32)  [unwired: 3 out]
              n256 = Array Max & Min(array=w712) -> (max index (indices)=w713:i32)  [unwired: 3 out]
              n257 = Index Array(array=w719, index=w718) -> (element=w709:string)
              n258 = Index Array(array=w711, index=w713) -> (element=w710:string)
            }
          }
        }
      }
    }
    frame "10224-1" {
      n259 = global read "Global_Cal Info.vi" "User Input_str"() -> (w777:string)
      n260 = case shown="\"\"" w777 {
        selector: w777 -> [w797 _]
        tunnel: [w797 w799] -> w776
        frame Default {
        }
        frame "" {
          n261 = call "User select_combobox.vi"("조합?"=FALSE, "문자열 입력"="0점 기준용 게이지 블록 치수는?", "배열 입력"=string[] ["6 mm", "11 mm"]) -> ("문자열 출력"=w800:string)  [unwired: 8 in]
          n262 = Search and Replace String(input string=w800, search string=" mm" ("검색 문자열")) -> (result string=w799:string)  [unwired: 6 in, 3 out]
        }
      }
      n263 = global write "Global_Cal Info.vi" "User Input_str"(w776) -> ()
      n264 = call "Create File Path.vi"("파일타입"=Cmd_File_Type."CSV", "항목"=Cmd_File_path."데이터파일경로", "에러 입력"=w772, "문자열 in"="Gauge Block Set_6" ("delimiter (\\t)")) -> ("error out"=w774:errorcluster, "파일경로"=w783:path)  [unwired: 4 in, 2 out]
      n265 = call-poly <vilib>:"Read Delimited Spreadsheet.vi"("file path (dialog if empty)"=w783, "error in (no error)"=w774, "delimiter (\\t)"="," ("delimiter (\\t)")) -> ("all rows"=w794:string[][], "error out"=w773:errorcluster)  [unwired: 7 in, 4 out]
      n266 = call-poly "Data Classification.vi"("인덱스"=2, "DATA 입력"=w794, "검색 문자열"=w776) -> ("DATA 출력"=w795:string[][])  [unwired: 4 in, 4 out]
      n267 = Index Array(array=w795, index (col) #1=0 ("비활성화된 인덱스 (열)")) -> (element #1=w785:string[], element #2=w786:string[])  [unwired: 3 in]
      n268 = Delete From Array(array=w795, length=5 ("길이"), index (col)=2 ("비활성화된 인덱스 (열)")) -> (deleted portion=w784:string[][])  [unwired: 1 in, 1 out]
      n269 = for {
        tunnel: w784 -> [w808]
        tunnel: w775 -> [w816]
        tunnel: w782 -> [w815] mode=indexing
        tunnel: w785 -> [w814]
        tunnel: w786 -> [w813]
        tunnel: w781 -> [w812] mode=indexing
        tunnel: [w811] -> w780 mode=indexing
        tunnel: [w810] -> w779 mode=indexing
        tunnel: [w804] -> w778
        n270 = for {
          tunnel: w815 -> [w832]
          tunnel: w812 -> [w831]
          tunnel: w808 -> [w828] mode=indexing
          tunnel: w816 -> [w818]
          tunnel: [w826] -> w811 if=w825
          tunnel: [w824] -> w810
          tunnel: w814 -> [w823] mode=indexing
          tunnel: w813 -> [w822] mode=indexing
          stop <- w825 stop-if-true
          n271 = Equal?(x=w832, y=w823) -> (x = y?=w829:bool)
          n272 = Equal?(x=w822, y=w831) -> (x = y?=w830:bool)
          n273 = Index Array(array=w818) -> (element=w820:string[])  [unwired: 2 in]
          n274 = Compound Arithmetic op=AND(w829, w830) -> (w827:bool)
          n275 = Delete From Array(array=w820, length=4 ("길이"), index=19 ("비활성화된 인덱스 (열)")) -> (deleted portion=w817:string[])  [unwired: 1 out]
          n276 = case shown="참" w827 {
            tunnel: w828 -> [_ w836]
            tunnel: [_ w838] -> w825
            tunnel: w818 -> [_ w837]
            tunnel: [_ w856] -> w826
            tunnel: [_ w851] -> w824
            tunnel: w817 -> [_ w841]
            frame False {
            }
            frame True {
              w844 = 0 ("인덱스")
              w852 = "Gauge Block" ("검색 문자열")
              n277 = call "Gauge Block Classification.vi"("블록삭제?(T)"=FALSE, "블록리스트"=w836, "게이지 블록 교정data"=w837) -> ("열팽창계수"=w833:string, "교정값(값)"=w839:dbl[], "블록치수"=w840:dbl[], "교정값(문자)"=w835:string[], "stop?"=w838:bool)  [unwired: 3 in, 1 out]
              n278 = Delete From Array(array=w840, index=w844) -> (deleted portion=w850:dbl, array with subset deleted=w846:dbl[])  [unwired: 1 in]
              n279 = Delete From Array(array=w839, index=w844) -> (deleted portion=w848:dbl, array with subset deleted=w845:dbl[])  [unwired: 1 in]
              n280 = Add Array Elements(numeric array=w846) -> (sum=w849:dbl)
              n281 = Add Array Elements(numeric array=w845) -> (sum=w847:dbl)
              n282 = Subtract(x=w849, y=w850) -> (x-y=w843:dbl)
              n283 = Subtract(x=w847, y=w848) -> (x-y=w842:dbl)
              n284 = Number To Fractional String(number=w843) -> (F-format string=w854:string)  [unwired: 3 in]
              n285 = Number To Fractional String(number=w842) -> (F-format string=w855:string)  [unwired: 3 in]
              n286 = Build Array (concatenate)(w852, w854, "mm" ("환산단위"), w855, w833, w841, w836, w835) -> (w856:string[])
              n287 = Build Array (concatenate)(w852, w836) -> (w851:string[])
            }
          }
        }
        n288 = for {
          tunnel: w808 -> [w858] mode=indexing
          tunnel: string[] ["0점블럭", "사용블럭#1", "사용블럭#2", "사용블럭#3", "사용블럭#4", "사용블럭#5"] -> [w859]
          tunnel: [w857] -> w805
          n289 = for {
            tunnel: w859 -> [w860] mode=indexing
            tunnel: w858 -> [_] mode=indexing
            tunnel: [w860] -> w857 mode=indexing
          }
        }
        n290 = Insert Into Array(array=w805, index=0 ("인덱스"), new element="기기명" ("새 원소/부분배열")) -> (w804:string[])
      }
    }
    frame "10232-1" {
      n291 = call-poly "Data Classification.vi"("인덱스"=2, "DATA 입력"=w866, "검색 문자열"="Gauge Block Accessory") -> ("DATA 출력"=w872:string[][])  [unwired: 4 in, 4 out]
      n292 = call "Variables Data IO.vi"("Write blank data ?(F)"=TRUE ("Write blank data ?(T)"), "Select"=Cmd_Var_Data_IO."STD4", "error in"=w864, "Data In"=w872, "Func_ext"=w868) -> ("error out"=w865:errorcluster)  [unwired: 4 in, 2 out]
      n293 = call "Create File Path.vi"("파일타입"=Cmd_File_Type."CSV", "항목"=Cmd_File_path."데이터파일경로", "에러 입력"=w865, "문자열 in"="Gauge Block Set_1" ("delimiter (\\t)")) -> ("error out"=w862:errorcluster, "파일경로"=w876:path)  [unwired: 4 in, 2 out]
      n294 = call-poly <vilib>:"Read Delimited Spreadsheet.vi"("file path (dialog if empty)"=w876, "error in (no error)"=w862, "delimiter (\\t)"="," ("delimiter (\\t)")) -> ("all rows"=w873:string[][], "error out"=w861:errorcluster)  [unwired: 7 in, 4 out]
      n295 = Index Array(array=w873, index (col) #1=0 ("비활성화된 인덱스 (열)")) -> (element #1=w888:string[], element #2=w889:string[])  [unwired: 3 in]
      n296 = Delete From Array(array=w873, length=5 ("길이"), index (col)=2 ("비활성화된 인덱스 (열)")) -> (deleted portion=w886:string[][])  [unwired: 1 in, 1 out]
      n297 = for {
        tunnel: w886 -> [w894]
        tunnel: w863 -> [w902]
        tunnel: w882 -> [w901] mode=indexing
        tunnel: w888 -> [w900]
        tunnel: w889 -> [w899]
        tunnel: w881 -> [w898] mode=indexing
        tunnel: [w897] -> w880 mode=indexing
        tunnel: [w896] -> w879 mode=indexing
        tunnel: [w892] -> w874
        n298 = case shown="기본" w901 {
          selector: w901 -> [_ w911]
          tunnel: w898 -> [_ w913]
          tunnel: w894 -> [_ w912]
          tunnel: w902 -> [_ w910]
          tunnel: [string[] ["Zero", "0"] w909] -> w897
          tunnel: [_ w908] -> w896
          tunnel: w900 -> [_ w907]
          tunnel: w899 -> [_ w906]
          frame "0" {
          }
          frame Default {
            n299 = for {
              tunnel: w911 -> [w932]
              tunnel: w913 -> [w931]
              tunnel: w912 -> [w928] mode=indexing
              tunnel: w910 -> [w918]
              tunnel: [w926] -> w909 if=w925
              tunnel: [w924] -> w908
              tunnel: w907 -> [w923] mode=indexing
              tunnel: w906 -> [w922] mode=indexing
              stop <- w925 stop-if-true
              w916 = 0 ("인덱스 (행)")
              n300 = Equal?(x=w932, y=w923) -> (x = y?=w929:bool)
              n301 = Equal?(x=w922, y=w931) -> (x = y?=w930:bool)
              n302 = Index Array(array=w918, index (row) #1=w916, index (col) #1=23 ("비활성화된 인덱스 (열)"), index (row) #2=w916) -> (element #1=w914:string, element #2=w920:string[])  [unwired: 1 in]
              n303 = Compound Arithmetic op=AND(w929, w930) -> (w927:bool)
              n304 = Delete From Array(array=w920, length=4 ("길이"), index=19 ("비활성화된 인덱스 (열)")) -> (deleted portion=w917:string[])  [unwired: 1 out]
              n305 = case shown="참" w927 {
                tunnel: w928 -> [_ w936]
                tunnel: [_ w940] -> w925
                tunnel: w918 -> [_ w937]
                tunnel: [_ w948] -> w926
                tunnel: [_ w942] -> w924
                tunnel: w917 -> [_ w941]
                tunnel: w914 -> [_ w935]
                frame False {
                }
                frame True {
                  w943 = "Gauge Block" ("검색 문자열")
                  n306 = call "Gauge Block Classification.vi"("블록리스트"=w936, "게이지 블록 교정data"=w937) -> ("열팽창계수"=w934:string, "교정값(값)"=w938:dbl[], "블록치수"=w939:dbl[], "교정값(문자)"=w933:string[], "stop?"=w940:bool)  [unwired: 4 in, 1 out]
                  n307 = Add Array Elements(numeric array=w939) -> (sum=w946:dbl)
                  n308 = Add Array Elements(numeric array=w938) -> (sum=w949:dbl)
                  n309 = Number To Fractional String(number=w946) -> (F-format string=w945:string)  [unwired: 3 in]
                  n310 = Number To Fractional String(number=w949) -> (F-format string=w947:string)  [unwired: 3 in]
                  n311 = Build Array (concatenate)(w943, w945, "mm" ("환산단위"), w947, w935, w934, w936, w933, w941) -> (w948:string[])
                  n312 = Build Array (concatenate)(w943, w936) -> (w942:string[])
                }
              }
            }
          }
        }
        n313 = Index Array(array=w894) -> (element=w895:string[])  [unwired: 2 in]
        n314 = for {
          tunnel: w895 -> [_] mode=indexing
          tunnel: [w903] -> w893 mode=indexing
          i -> [w904]
          n315 = Format Into String(w904) -> (resulting string=w903:string)  [unwired: 3 in, 1 out]
        }
        n316 = Replace Array Subset(array=w893, new element="기기명" ("새 원소/부분배열"), index=0 ("인덱스")) -> (w892:string[])
      }
    }
    frame "10232-2" {
      n317 = call-poly "Data Classification.vi"("인덱스"=2, "DATA 입력"=w957, "검색 문자열"="Gauge Block Accessory") -> ("DATA 출력"=w963:string[][])  [unwired: 4 in, 4 out]
      n318 = call "Variables Data IO.vi"("Write blank data ?(F)"=TRUE ("Write blank data ?(T)"), "Select"=Cmd_Var_Data_IO."STD4", "error in"=w955, "Data In"=w963, "Func_ext"=w959) -> ("error out"=w956:errorcluster)  [unwired: 4 in, 2 out]
      n319 = call "Create File Path.vi"("파일타입"=Cmd_File_Type."CSV", "항목"=Cmd_File_path."데이터파일경로", "에러 입력"=w956, "문자열 in"="Gauge Block Set_1" ("delimiter (\\t)")) -> ("error out"=w953:errorcluster, "파일경로"=w967:path)  [unwired: 4 in, 2 out]
      n320 = call-poly <vilib>:"Read Delimited Spreadsheet.vi"("file path (dialog if empty)"=w967, "error in (no error)"=w953, "delimiter (\\t)"="," ("delimiter (\\t)")) -> ("all rows"=w964:string[][], "error out"=w952:errorcluster)  [unwired: 7 in, 4 out]
      n321 = Index Array(array=w964, index (col) #1=0 ("비활성화된 인덱스 (열)")) -> (element #1=w977:string[], element #2=w978:string[])  [unwired: 3 in]
      n322 = Delete From Array(array=w964, length=5 ("길이"), index (col)=2 ("비활성화된 인덱스 (열)")) -> (deleted portion=w975:string[][])  [unwired: 1 in, 1 out]
      n323 = for {
        tunnel: w975 -> [w983]
        tunnel: w954 -> [w991]
        tunnel: w951 -> [w990] mode=indexing
        tunnel: w977 -> [w989]
        tunnel: w978 -> [w988]
        tunnel: w950 -> [w987] mode=indexing
        tunnel: [w986] -> w971 mode=indexing
        tunnel: [w985] -> w970 mode=indexing
        tunnel: [w981] -> w965
        n324 = case shown="기본" w990 {
          selector: w990 -> [_ w1000]
          tunnel: w987 -> [_ w1002]
          tunnel: w983 -> [_ w1001]
          tunnel: w991 -> [_ w999]
          tunnel: [string[] ["Zero", "0"] w998] -> w986
          tunnel: [_ w997] -> w985
          tunnel: w989 -> [_ w996]
          tunnel: w988 -> [_ w995]
          frame "0" {
          }
          frame Default {
            n325 = for {
              tunnel: w1000 -> [w1021]
              tunnel: w1002 -> [w1020]
              tunnel: w1001 -> [w1017] mode=indexing
              tunnel: w999 -> [w1007]
              tunnel: [w1015] -> w998 if=w1014
              tunnel: [w1013] -> w997
              tunnel: w996 -> [w1012] mode=indexing
              tunnel: w995 -> [w1011] mode=indexing
              stop <- w1014 stop-if-true
              w1005 = 0 ("인덱스 (행)")
              n326 = Equal?(x=w1021, y=w1012) -> (x = y?=w1018:bool)
              n327 = Equal?(x=w1011, y=w1020) -> (x = y?=w1019:bool)
              n328 = Index Array(array=w1007, index (row) #1=w1005, index (col) #1=23 ("비활성화된 인덱스 (열)"), index (row) #2=w1005) -> (element #1=w1003:string, element #2=w1009:string[])  [unwired: 1 in]
              n329 = Compound Arithmetic op=AND(w1018, w1019) -> (w1016:bool)
              n330 = Delete From Array(array=w1009, length=4 ("길이"), index=19 ("비활성화된 인덱스 (열)")) -> (deleted portion=w1006:string[])  [unwired: 1 out]
              n331 = case shown="참" w1016 {
                tunnel: w1017 -> [_ w1025]
                tunnel: [_ w1029] -> w1014
                tunnel: w1007 -> [_ w1026]
                tunnel: [_ w1037] -> w1015
                tunnel: [_ w1031] -> w1013
                tunnel: w1006 -> [_ w1030]
                tunnel: w1003 -> [_ w1024]
                frame False {
                }
                frame True {
                  w1032 = "Gauge Block" ("검색 문자열")
                  n332 = call "Gauge Block Classification.vi"("블록리스트"=w1025, "게이지 블록 교정data"=w1026) -> ("열팽창계수"=w1023:string, "교정값(값)"=w1027:dbl[], "블록치수"=w1028:dbl[], "교정값(문자)"=w1022:string[], "stop?"=w1029:bool)  [unwired: 4 in, 1 out]
                  n333 = Add Array Elements(numeric array=w1028) -> (sum=w1035:dbl)
                  n334 = Add Array Elements(numeric array=w1027) -> (sum=w1038:dbl)
                  n335 = Number To Fractional String(number=w1035) -> (F-format string=w1034:string)  [unwired: 3 in]
                  n336 = Number To Fractional String(number=w1038) -> (F-format string=w1036:string)  [unwired: 3 in]
                  n337 = Build Array (concatenate)(w1032, w1034, "mm" ("환산단위"), w1036, w1024, w1023, w1025, w1022, w1030) -> (w1037:string[])
                  n338 = Build Array (concatenate)(w1032, w1025) -> (w1031:string[])
                }
              }
            }
          }
        }
        n339 = Index Array(array=w983) -> (element=w984:string[])  [unwired: 2 in]
        n340 = for {
          tunnel: w984 -> [_] mode=indexing
          tunnel: [w992] -> w982 mode=indexing
          i -> [w993]
          n341 = Format Into String(w993) -> (resulting string=w992:string)  [unwired: 3 in, 1 out]
        }
        n342 = Replace Array Subset(array=w982, new element="기기명" ("새 원소/부분배열"), index=0 ("인덱스")) -> (w981:string[])
      }
    }
    frame "10235-2", "10605-1", "10605-2" {
      n343 = call "Create File Path.vi"("파일타입"=Cmd_File_Type."CSV", "항목"=Cmd_File_path."데이터파일경로", "에러 입력"=w1048, "문자열 in"="Gauge Block Set_2" ("delimiter (\\t)")) -> ("error out"=w1040:errorcluster, "파일경로"=w1045:path)  [unwired: 4 in, 2 out]
      n344 = call-poly <vilib>:"Read Delimited Spreadsheet.vi"("file path (dialog if empty)"=w1045, "error in (no error)"=w1040, "delimiter (\\t)"="," ("delimiter (\\t)")) -> ("all rows"=w1042:string[][], "error out"=w1039:errorcluster)  [unwired: 7 in, 4 out]
      n345 = Index Array(array=w1042, index (col) #1=0 ("비활성화된 인덱스 (열)")) -> (element #1=w1058:string[], element #2=w1059:string[])  [unwired: 3 in]
      n346 = Delete From Array(array=w1042, length=5 ("길이"), index (col)=2 ("비활성화된 인덱스 (열)")) -> (deleted portion=w1056:string[][])  [unwired: 1 in, 1 out]
      n347 = for {
        tunnel: w1056 -> [w1064]
        tunnel: w1041 -> [w1072]
        tunnel: w1052 -> [w1071] mode=indexing
        tunnel: w1058 -> [w1070]
        tunnel: w1059 -> [w1069]
        tunnel: w1051 -> [w1068] mode=indexing
        tunnel: [w1067] -> w1050 mode=indexing
        tunnel: [w1066] -> w1049 mode=indexing
        tunnel: [w1060] -> w1043
        n348 = case shown="기본" w1071 {
          selector: w1071 -> [_ w1083]
          tunnel: w1068 -> [_ w1085]
          tunnel: w1064 -> [_ w1084]
          tunnel: w1072 -> [_ w1082]
          tunnel: [string[] ["Gauge Block", "0"] w1081] -> w1067
          tunnel: [_ w1080] -> w1066
          tunnel: w1070 -> [_ w1079]
          tunnel: w1069 -> [_ w1078]
          frame "0" {
          }
          frame Default {
            n349 = for {
              tunnel: w1083 -> [w1104]
              tunnel: w1085 -> [w1103]
              tunnel: w1084 -> [w1100] mode=indexing
              tunnel: w1082 -> [w1090]
              tunnel: [w1098] -> w1081 if=w1097
              tunnel: [w1096] -> w1080
              tunnel: w1079 -> [w1095] mode=indexing
              tunnel: w1078 -> [w1094] mode=indexing
              stop <- w1097 stop-if-true
              n350 = Equal?(x=w1104, y=w1095) -> (x = y?=w1101:bool)
              n351 = Equal?(x=w1094, y=w1103) -> (x = y?=w1102:bool)
              n352 = Index Array(array=w1090, index (row) #2=0 ("인덱스 (행)"), index (col) #2=23 ("비활성화된 인덱스 (열)")) -> (element #1=w1092:string[], element #2=w1086:string)  [unwired: 2 in]
              n353 = Compound Arithmetic op=AND(w1101, w1102) -> (w1099:bool)
              n354 = Delete From Array(array=w1092, length=4 ("길이"), index=19 ("비활성화된 인덱스 (열)")) -> (deleted portion=w1089:string[])  [unwired: 1 out]
              n355 = case shown="참" w1099 {
                tunnel: w1100 -> [_ w1109]
                tunnel: [_ w1111] -> w1097
                tunnel: w1090 -> [_ w1110]
                tunnel: [_ w1128] -> w1098
                tunnel: [_ w1124] -> w1096
                tunnel: w1089 -> [_ w1114]
                tunnel: w1086 -> [_ w1108]
                frame False {
                }
                frame True {
                  w1117 = 0 ("인덱스")
                  w1105 = "mm" ("환산단위")
                  w1125 = "Gauge Block" ("검색 문자열")
                  n356 = call "Gauge Block Classification.vi"("블록리스트"=w1109, "게이지 블록 교정data"=w1110) -> ("열팽창계수"=w1107:string, "교정값(값)"=w1112:dbl[], "블록치수"=w1113:dbl[], "교정값(문자)"=w1106:string[], "stop?"=w1111:bool)  [unwired: 4 in, 1 out]
                  n357 = Delete From Array(array=w1113, index=w1117) -> (deleted portion=w1123:dbl, array with subset deleted=w1119:dbl[])  [unwired: 1 in]
                  n358 = Delete From Array(array=w1112, index=w1117) -> (deleted portion=w1121:dbl, array with subset deleted=w1118:dbl[])  [unwired: 1 in]
                  n359 = Add Array Elements(numeric array=w1119) -> (sum=w1122:dbl)
                  n360 = Add Array Elements(numeric array=w1118) -> (sum=w1120:dbl)
                  n361 = Subtract(x=w1122, y=w1123) -> (x-y=w1116:dbl)
                  n362 = Subtract(x=w1120, y=w1121) -> (x-y=w1115:dbl)
                  n363 = Number To Fractional String(number=w1116) -> (F-format string=w1126:string)  [unwired: 3 in]
                  n364 = Number To Fractional String(number=w1115) -> (F-format string=w1127:string)  [unwired: 3 in]
                  n365 = Build Array (concatenate)(w1125, w1126, w1105, w1127, w1105, w1114, w1108, w1107, w1109, w1106) -> (w1128:string[])
                  n366 = Build Array (concatenate)(w1125, w1109) -> (w1124:string[])
                }
              }
            }
          }
        }
        n367 = for {
          tunnel: w1064 -> [w1074] mode=indexing
          tunnel: string[] ["0점블럭", "사용블럭#1", "사용블럭#2", "사용블럭#3", "사용블럭#4", "사용블럭#5"] -> [w1075]
          tunnel: [w1073] -> w1061
          n368 = for {
            tunnel: w1075 -> [w1076] mode=indexing
            tunnel: w1074 -> [_] mode=indexing
            tunnel: [w1076] -> w1073 mode=indexing
          }
        }
        n369 = Insert Into Array(array=w1061, index=0 ("인덱스"), new element="기기명" ("새 원소/부분배열")) -> (w1060:string[])
      }
    }
    frame "10604-1", "10604-2" {
      n370 = call "Create File Path.vi"("파일타입"=Cmd_File_Type."CSV", "항목"=Cmd_File_path."데이터파일경로", "에러 입력"=w1138, "문자열 in"="Gauge Block Set_3" ("delimiter (\\t)")) -> ("error out"=w1130:errorcluster, "파일경로"=w1135:path)  [unwired: 4 in, 2 out]
      n371 = call-poly <vilib>:"Read Delimited Spreadsheet.vi"("file path (dialog if empty)"=w1135, "error in (no error)"=w1130, "delimiter (\\t)"="," ("delimiter (\\t)")) -> ("all rows"=w1132:string[][], "error out"=w1129:errorcluster)  [unwired: 7 in, 4 out]
      n372 = Index Array(array=w1132, index (col) #1=0 ("비활성화된 인덱스 (열)")) -> (element #1=w1148:string[], element #2=w1149:string[])  [unwired: 3 in]
      n373 = Delete From Array(array=w1132, length=12 ("길이"), index (col)=2 ("비활성화된 인덱스 (열)")) -> (deleted portion=w1146:string[][])  [unwired: 1 in, 1 out]
      n374 = for {
        tunnel: w1146 -> [w1151]
        tunnel: w1131 -> [w1159]
        tunnel: w1142 -> [w1158] mode=indexing
        tunnel: w1148 -> [w1157]
        tunnel: w1149 -> [w1156]
        tunnel: w1141 -> [w1155] mode=indexing
        tunnel: [w1154] -> w1140 mode=indexing
        tunnel: [w1153] -> w1139 mode=indexing
        tunnel: [w1150] -> w1133
        n375 = case shown="기본" w1158 {
          selector: w1158 -> [_ w1170]
          tunnel: w1155 -> [_ w1172]
          tunnel: w1151 -> [_ w1171]
          tunnel: w1159 -> [_ w1169]
          tunnel: [string[] ["Gauge Block", "0"] w1168] -> w1154
          tunnel: [_ w1167] -> w1153
          tunnel: w1157 -> [_ w1166]
          tunnel: w1156 -> [_ w1165]
          frame "0" {
          }
          frame Default {
            n376 = for {
              tunnel: w1170 -> [w1177]
              tunnel: w1172 -> [w1190]
              tunnel: w1171 -> [w1187] mode=indexing
              tunnel: w1169 -> [w1176]
              tunnel: [w1185] -> w1168 if=w1184
              tunnel: [w1183] -> w1167
              tunnel: w1166 -> [w1182] mode=indexing
              tunnel: w1165 -> [w1181] mode=indexing
              stop <- w1184 stop-if-true
              n377 = Equal?(x=w1177, y=w1182) -> (x = y?=w1188:bool)
              n378 = Equal?(x=w1181, y=w1190) -> (x = y?=w1189:bool)
              n379 = Compound Arithmetic op=AND(w1188, w1189) -> (w1186:bool)
              n380 = Delete From Array(array=w1176, length=4 ("길이"), index (col)=19 ("비활성화된 인덱스 (열)")) -> (deleted portion=w1178:string[][])  [unwired: 1 in, 1 out]
              n381 = Index Array(array=w1176, index (row)=0 ("인덱스 (행)"), index (col)=23 ("비활성화된 인덱스 (열)")) -> (element=w1173:string)
              n382 = case shown="참" w1186 {
                tunnel: w1187 -> [_ w1225]
                tunnel: [_ w1232] -> w1184
                tunnel: w1176 -> [_ w1234]
                tunnel: [_ w1233] -> w1185
                tunnel: [_ w1225] -> w1183
                tunnel: w1178 -> [_ w1203]
                tunnel: w1177 -> [_ w1202]
                tunnel: w1173 -> [_ w1195]
                frame False {
                }
                frame True {
                  w1191 = "mm" ("원소")
                  w1220 = 4 ("길이")
                  n383 = call-poly "Array Deduplication.vi"("배열 in"=w1203) -> ("배열 out"=w1200:string[][])  [unwired: 9 in, 1 out]
                  n384 = Fract/Exp String To Number(string=w1202) -> (number=w1201:dbl)  [unwired: 3 in, 1 out]
                  n385 = call "Gauge Block Classification.vi"("블록리스트"=w1225, "게이지 블록 교정data"=w1234) -> ("열팽창계수"=w1194:string, "교정값(값)"=w1219:dbl[], "블록치수"=w1226:dbl[], "교정값(문자)"=w1193:string[], "stop?"=w1232:bool)  [unwired: 4 in, 1 out]
                  n386 = for {
                    tunnel: w1200 -> [w1235] mode=indexing
                    tunnel: w1201 -> [w1243]
                    tunnel: [w1236] -> w1199 mode=indexing
                    tunnel: [w1235] -> w1198 mode=indexing
                    n387 = Fract/Exp String To Number(string=w1235) -> (number=w1244:dbl[])  [unwired: 3 in, 1 out]
                    n388 = Index Array(array=w1244) -> (element #1=w1241:dbl, element #2=w1242:dbl)  [unwired: 2 in]
                    n389 = Multiply(x=w1242, y=w1243) -> (x*y=w1240:dbl)
                    n390 = Square(x=w1241) -> (x^2=w1239:dbl)
                    n391 = Square(x=w1240) -> (x^2=w1238:dbl)
                    n392 = Add(x=w1239, y=w1238) -> (x+y=w1237:dbl)
                    n393 = Square Root(x=w1237) -> (sqrt(x)=w1236:dbl)
                  }
                  n394 = Delete From Array(array=w1226, length=w1220) -> (deleted portion=w1230:dbl[], array with subset deleted=w1231:dbl[])  [unwired: 1 in]
                  n395 = Delete From Array(array=w1219, length=w1220) -> (deleted portion=w1222:dbl[], array with subset deleted=w1221:dbl[])  [unwired: 1 in]
                  n396 = Delete From Array(array=w1231, length=w1220) -> (deleted portion=w1228:dbl[], array with subset deleted=w1229:dbl[])  [unwired: 1 in]
                  n397 = Delete From Array(array=w1221, length=w1220) -> (deleted portion=w1224:dbl[], array with subset deleted=w1223:dbl[])  [unwired: 1 in]
                  n398 = Add Array Elements(numeric array=w1229) -> (sum=w1217:dbl)
                  n399 = Add Array Elements(numeric array=w1228) -> (sum=w1216:dbl)
                  n400 = Add Array Elements(numeric array=w1230) -> (sum=w1211:dbl)
                  n401 = Add Array Elements(numeric array=w1223) -> (sum=w1206:dbl)
                  n402 = Add Array Elements(numeric array=w1224) -> (sum=w1207:dbl)
                  n403 = Add Array Elements(numeric array=w1222) -> (sum=w1205:dbl)
                  n404 = Add(x=w1217, y=w1216) -> (x+y=w1215:dbl)
                  n405 = Add(x=w1206, y=w1207) -> (x+y=w1208:dbl)
                  n406 = Array Max & Min(array=w1199) -> (max index (indices)=w1197:i32)  [unwired: 3 out]
                  n407 = Divide(x=w1215, y=2.0) -> (x/y=w1213:dbl)
                  n408 = Divide(x=w1208, y=2.0) -> (x/y=w1210:dbl)
                  n409 = Subtract(x=w1213, y=w1211) -> (x-y=w1212:dbl)
                  n410 = Subtract(x=w1210, y=w1205) -> (x-y=w1204:dbl)
                  n411 = Index Array(array=w1198, index (row)=w1197) -> (element=w1196:string[])  [unwired: 1 in]
                  n412 = Number To Fractional String(number=w1212) -> (F-format string=w1227:string)  [unwired: 3 in]
                  n413 = Number To Fractional String(number=w1204) -> (F-format string=w1218:string)  [unwired: 3 in]
                  n414 = Build Array (concatenate)("Gauge Block" ("검색 문자열"), w1227, w1191, w1218, w1191, w1196, w1195, w1194, w1225, w1193) -> (w1233:string[])
                }
              }
            }
          }
        }
        n415 = for {
          tunnel: w1151 -> [w1161] mode=indexing
          tunnel: string[] ["L블럭#1", "L블럭#2", "L블럭#3", "L블럭#4", "R블럭#1", "R블럭#2", "R블럭#3", "R블럭#4", "Center#1", "Center#2", "Center#3", "Center#4"] -> [w1162]
          tunnel: [w1160] -> w1150
          n416 = for {
            tunnel: w1162 -> [w1163] mode=indexing
            tunnel: w1161 -> [_] mode=indexing
            tunnel: [w1163] -> w1160 mode=indexing
          }
        }
      }
    }
    frame "10613-1" {
      n417 = call-poly "Data Classification.vi"("인덱스"=2, "DATA 입력"=w1250, "검색 문자열"="Gauge Block Accessory") -> ("DATA 출력"=w1256:string[][])  [unwired: 4 in, 4 out]
      n418 = call "Variables Data IO.vi"("Write blank data ?(F)"=TRUE ("Write blank data ?(T)"), "Select"=Cmd_Var_Data_IO."STD2", "error in"=w1248, "Data In"=w1256, "Func_ext"=w1252) -> ("error out"=w1249:errorcluster)  [unwired: 4 in, 2 out]
      n419 = call "Create File Path.vi"("파일타입"=Cmd_File_Type."CSV", "항목"=Cmd_File_path."데이터파일경로", "에러 입력"=w1249, "문자열 in"="Gauge Block Set_1" ("delimiter (\\t)")) -> ("error out"=w1246:errorcluster, "파일경로"=w1260:path)  [unwired: 4 in, 2 out]
      n420 = call-poly <vilib>:"Read Delimited Spreadsheet.vi"("file path (dialog if empty)"=w1260, "error in (no error)"=w1246, "delimiter (\\t)"="," ("delimiter (\\t)")) -> ("all rows"=w1257:string[][], "error out"=w1245:errorcluster)  [unwired: 7 in, 4 out]
      n421 = Index Array(array=w1257, index (col) #1=0 ("비활성화된 인덱스 (열)")) -> (element #1=w1272:string[], element #2=w1273:string[])  [unwired: 3 in]
      n422 = Delete From Array(array=w1257, length=5 ("길이"), index (col)=2 ("비활성화된 인덱스 (열)")) -> (deleted portion=w1270:string[][])  [unwired: 1 in, 1 out]
      n423 = for {
        tunnel: w1270 -> [w1278]
        tunnel: w1247 -> [w1286]
        tunnel: w1266 -> [w1285] mode=indexing
        tunnel: w1272 -> [w1284]
        tunnel: w1273 -> [w1283]
        tunnel: w1265 -> [w1282] mode=indexing
        tunnel: [w1281] -> w1264 mode=indexing
        tunnel: [w1280] -> w1263 mode=indexing
        tunnel: [w1276] -> w1258
        n424 = case shown="기본" w1285 {
          selector: w1285 -> [_ w1295]
          tunnel: w1282 -> [_ w1297]
          tunnel: w1278 -> [_ w1296]
          tunnel: w1286 -> [_ w1294]
          tunnel: [string[] ["Zero", "0"] w1293] -> w1281
          tunnel: [_ w1292] -> w1280
          tunnel: w1284 -> [_ w1291]
          tunnel: w1283 -> [_ w1290]
          frame "0" {
          }
          frame Default {
            n425 = for {
              tunnel: w1295 -> [w1309]
              tunnel: w1297 -> [w1308]
              tunnel: w1296 -> [w1305] mode=indexing
              tunnel: w1294 -> [w1298]
              tunnel: [w1303] -> w1293 if=w1302
              tunnel: [w1301] -> w1292
              tunnel: w1291 -> [w1300] mode=indexing
              tunnel: w1290 -> [w1299] mode=indexing
              stop <- w1302 stop-if-true
              n426 = Equal?(x=w1309, y=w1300) -> (x = y?=w1306:bool)
              n427 = Equal?(x=w1299, y=w1308) -> (x = y?=w1307:bool)
              n428 = Compound Arithmetic op=AND(w1306, w1307) -> (w1304:bool)
              n429 = case shown="참" w1304 {
                tunnel: w1305 -> [_ w1313]
                tunnel: [_ w1317] -> w1302
                tunnel: w1298 -> [_ w1314]
                tunnel: [_ w1324] -> w1303
                tunnel: [_ w1318] -> w1301
                frame False {
                }
                frame True {
                  w1319 = "Gauge Block" ("검색 문자열")
                  n430 = call "Gauge Block Classification.vi"("블록리스트"=w1313, "게이지 블록 교정data"=w1314) -> ("불확도배열"=w1310:string[], "열팽창계수"=w1311:string, "교정값(값)"=w1315:dbl[], "블록치수"=w1316:dbl[], "교정값(문자)"=w1312:string[], "stop?"=w1317:bool)  [unwired: 4 in]
                  n431 = Add Array Elements(numeric array=w1316) -> (sum=w1322:dbl)
                  n432 = Add Array Elements(numeric array=w1315) -> (sum=w1325:dbl)
                  n433 = Number To Fractional String(number=w1322) -> (F-format string=w1321:string)  [unwired: 3 in]
                  n434 = Number To Fractional String(number=w1325) -> (F-format string=w1323:string)  [unwired: 3 in]
                  n435 = Build Array (concatenate)(w1319, w1321, "mm" ("환산단위"), w1323, w1313, w1312, w1311, w1310) -> (w1324:string[])
                  n436 = Build Array (concatenate)(w1319, w1313) -> (w1318:string[])
                }
              }
            }
          }
        }
        n437 = Index Array(array=w1278) -> (element=w1279:string[])  [unwired: 2 in]
        n438 = for {
          tunnel: w1279 -> [_] mode=indexing
          tunnel: [w1287] -> w1277 mode=indexing
          i -> [w1288]
          n439 = Format Into String(w1288) -> (resulting string=w1287:string)  [unwired: 3 in, 1 out]
        }
        n440 = Replace Array Subset(array=w1277, new element="기기명" ("새 원소/부분배열"), index=0 ("인덱스")) -> (w1276:string[])
      }
    }
    frame Default {
      n441 = call-poly "Data Classification.vi"("인덱스"=2, "DATA 입력"=w1331, "검색 문자열"="Gauge Block Accessory") -> ("DATA 출력"=w1337:string[][])  [unwired: 4 in, 4 out]
      n442 = call "Variables Data IO.vi"("Write blank data ?(F)"=TRUE ("Write blank data ?(T)"), "Select"=Cmd_Var_Data_IO."STD2", "error in"=w1329, "Data In"=w1337, "Func_ext"=w1333) -> ("error out"=w1330:errorcluster)  [unwired: 4 in, 2 out]
      n443 = call "Create File Path.vi"("파일타입"=Cmd_File_Type."CSV", "항목"=Cmd_File_path."데이터파일경로", "에러 입력"=w1330, "문자열 in"="Gauge Block Set_1" ("delimiter (\\t)")) -> ("error out"=w1327:errorcluster, "파일경로"=w1341:path)  [unwired: 4 in, 2 out]
      n444 = call-poly <vilib>:"Read Delimited Spreadsheet.vi"("file path (dialog if empty)"=w1341, "error in (no error)"=w1327, "delimiter (\\t)"="," ("delimiter (\\t)")) -> ("all rows"=w1338:string[][], "error out"=w1326:errorcluster)  [unwired: 7 in, 4 out]
      n445 = Index Array(array=w1338, index (col) #1=0 ("비활성화된 인덱스 (열)")) -> (element #1=w1353:string[], element #2=w1354:string[])  [unwired: 3 in]
      n446 = Delete From Array(array=w1338, length=5 ("길이"), index (col)=2 ("비활성화된 인덱스 (열)")) -> (deleted portion=w1351:string[][])  [unwired: 1 in, 1 out]
      n447 = for {
        tunnel: w1351 -> [w1359]
        tunnel: w1328 -> [w1367]
        tunnel: w1347 -> [w1366] mode=indexing
        tunnel: w1353 -> [w1365]
        tunnel: w1354 -> [w1364]
        tunnel: w1346 -> [w1363] mode=indexing
        tunnel: [w1362] -> w1345 mode=indexing
        tunnel: [w1361] -> w1344 mode=indexing
        tunnel: [w1357] -> w1339
        n448 = case shown="기본" w1366 {
          selector: w1366 -> [_ w1376]
          tunnel: w1363 -> [_ w1378]
          tunnel: w1359 -> [_ w1377]
          tunnel: w1367 -> [_ w1375]
          tunnel: [string[] ["Zero", "0"] w1374] -> w1362
          tunnel: [_ w1373] -> w1361
          tunnel: w1365 -> [_ w1372]
          tunnel: w1364 -> [_ w1371]
          frame "0" {
          }
          frame Default {
            n449 = for {
              tunnel: w1376 -> [w1397]
              tunnel: w1378 -> [w1396]
              tunnel: w1377 -> [w1393] mode=indexing
              tunnel: w1375 -> [w1383]
              tunnel: [w1391] -> w1374 if=w1390
              tunnel: [w1389] -> w1373
              tunnel: w1372 -> [w1388] mode=indexing
              tunnel: w1371 -> [w1387] mode=indexing
              stop <- w1390 stop-if-true
              w1381 = 0 ("인덱스 (행)")
              n450 = Equal?(x=w1397, y=w1388) -> (x = y?=w1394:bool)
              n451 = Equal?(x=w1387, y=w1396) -> (x = y?=w1395:bool)
              n452 = Index Array(array=w1383, index (row) #1=w1381, index (col) #1=23 ("비활성화된 인덱스 (열)"), index (row) #2=w1381) -> (element #1=w1379:string, element #2=w1385:string[])  [unwired: 1 in]
              n453 = Compound Arithmetic op=AND(w1394, w1395) -> (w1392:bool)
              n454 = Delete From Array(array=w1385, length=4 ("길이"), index=19 ("비활성화된 인덱스 (열)")) -> (deleted portion=w1382:string[])  [unwired: 1 out]
              n455 = case shown="참" w1392 {
                tunnel: w1393 -> [_ w1401]
                tunnel: [_ w1405] -> w1390
                tunnel: w1383 -> [_ w1402]
                tunnel: [_ w1413] -> w1391
                tunnel: [_ w1407] -> w1389
                tunnel: w1382 -> [_ w1406]
                tunnel: w1379 -> [_ w1400]
                frame False {
                }
                frame True {
                  w1408 = "Gauge Block" ("검색 문자열")
                  n456 = call "Gauge Block Classification.vi"("블록리스트"=w1401, "게이지 블록 교정data"=w1402) -> ("열팽창계수"=w1399:string, "교정값(값)"=w1403:dbl[], "블록치수"=w1404:dbl[], "교정값(문자)"=w1398:string[], "stop?"=w1405:bool)  [unwired: 4 in, 1 out]
                  n457 = Add Array Elements(numeric array=w1404) -> (sum=w1411:dbl)
                  n458 = Add Array Elements(numeric array=w1403) -> (sum=w1414:dbl)
                  n459 = Number To Fractional String(number=w1411) -> (F-format string=w1410:string)  [unwired: 3 in]
                  n460 = Number To Fractional String(number=w1414) -> (F-format string=w1412:string)  [unwired: 3 in]
                  n461 = Build Array (concatenate)(w1408, w1410, "mm" ("환산단위"), w1412, w1400, w1399, w1401, w1398, w1406) -> (w1413:string[])
                  n462 = Build Array (concatenate)(w1408, w1401) -> (w1407:string[])
                }
              }
            }
          }
        }
        n463 = Index Array(array=w1359) -> (element=w1360:string[])  [unwired: 2 in]
        n464 = for {
          tunnel: w1360 -> [_] mode=indexing
          tunnel: [w1368] -> w1358 mode=indexing
          i -> [w1369]
          n465 = Format Into String(w1369) -> (resulting string=w1368:string)  [unwired: 3 in, 1 out]
        }
        n466 = Replace Array Subset(array=w1358, new element="기기명" ("새 원소/부분배열"), index=0 ("인덱스")) -> (w1357:string[])
      }
    }
    frame "10503-0" {
      n467 = call-poly "Data Classification.vi"("인덱스"=2, "DATA 입력"=w1420, "검색 문자열"="Gauge Block Accessory") -> ("DATA 출력"=w1426:string[][])  [unwired: 4 in, 4 out]
      n468 = call "Variables Data IO.vi"("Write blank data ?(F)"=TRUE ("Write blank data ?(T)"), "Select"=Cmd_Var_Data_IO."STD2", "error in"=w1418, "Data In"=w1426, "Func_ext"=w1422) -> ("error out"=w1419:errorcluster)  [unwired: 4 in, 2 out]
      n469 = call "Create File Path.vi"("파일타입"=Cmd_File_Type."CSV", "항목"=Cmd_File_path."데이터파일경로", "에러 입력"=w1419, "문자열 in"="Gauge Block Set_1" ("delimiter (\\t)")) -> ("error out"=w1416:errorcluster, "파일경로"=w1430:path)  [unwired: 4 in, 2 out]
      n470 = call-poly <vilib>:"Read Delimited Spreadsheet.vi"("file path (dialog if empty)"=w1430, "error in (no error)"=w1416, "delimiter (\\t)"="," ("delimiter (\\t)")) -> ("all rows"=w1427:string[][], "error out"=w1415:errorcluster)  [unwired: 7 in, 4 out]
      n471 = Index Array(array=w1427, index (col) #1=0 ("비활성화된 인덱스 (열)")) -> (element #1=w1442:string[], element #2=w1443:string[])  [unwired: 3 in]
      n472 = Delete From Array(array=w1427, length=5 ("길이"), index (col)=2 ("비활성화된 인덱스 (열)")) -> (deleted portion=w1440:string[][])  [unwired: 1 in, 1 out]
      n473 = for {
        tunnel: w1440 -> [w1448]
        tunnel: w1417 -> [w1456]
        tunnel: w1436 -> [w1455] mode=indexing
        tunnel: w1442 -> [w1454]
        tunnel: w1443 -> [w1453]
        tunnel: w1435 -> [w1452] mode=indexing
        tunnel: [w1451] -> w1434 mode=indexing
        tunnel: [w1450] -> w1433 mode=indexing
        tunnel: [w1446] -> w1428
        n474 = case shown="기본" w1455 {
          selector: w1455 -> [_ w1465]
          tunnel: w1452 -> [_ w1467]
          tunnel: w1448 -> [_ w1466]
          tunnel: w1456 -> [_ w1464]
          tunnel: [string[] ["Zero", "0"] w1463] -> w1451
          tunnel: [_ w1462] -> w1450
          tunnel: w1454 -> [_ w1461]
          tunnel: w1453 -> [_ w1460]
          frame "0" {
          }
          frame Default {
            n475 = for {
              tunnel: w1465 -> [w1486]
              tunnel: w1467 -> [w1485]
              tunnel: w1466 -> [w1482] mode=indexing
              tunnel: w1464 -> [w1472]
              tunnel: [w1480] -> w1463 if=w1479
              tunnel: [w1478] -> w1462
              tunnel: w1461 -> [w1477] mode=indexing
              tunnel: w1460 -> [w1476] mode=indexing
              stop <- w1479 stop-if-true
              w1470 = 0 ("인덱스 (행)")
              n476 = Equal?(x=w1486, y=w1477) -> (x = y?=w1483:bool)
              n477 = Equal?(x=w1476, y=w1485) -> (x = y?=w1484:bool)
              n478 = Index Array(array=w1472, index (row) #1=w1470, index (col) #1=23 ("비활성화된 인덱스 (열)"), index (row) #2=w1470) -> (element #1=w1468:string, element #2=w1474:string[])  [unwired: 1 in]
              n479 = Compound Arithmetic op=AND(w1483, w1484) -> (w1481:bool)
              n480 = Delete From Array(array=w1474, length=4 ("길이"), index=19 ("비활성화된 인덱스 (열)")) -> (deleted portion=w1471:string[])  [unwired: 1 out]
              n481 = case shown="참" w1481 {
                tunnel: w1482 -> [_ w1490]
                tunnel: [_ w1494] -> w1479
                tunnel: w1472 -> [_ w1491]
                tunnel: [_ w1501] -> w1480
                tunnel: [_ w1496] -> w1478
                tunnel: w1471 -> [_ w1495]
                tunnel: w1468 -> [_ w1488]
                frame False {
                }
                frame True {
                  w1489 = "mm" ("환산단위")
                  w1497 = "Gauge Block" ("검색 문자열")
                  n482 = call "Gauge Block Classification.vi"("블록리스트"=w1490, "게이지 블록 교정data"=w1491) -> ("열팽창계수"=w1487:string, "교정값(값)"=w1492:dbl[], "블록치수"=w1493:dbl[], "stop?"=w1494:bool)  [unwired: 4 in, 2 out]
                  n483 = Add Array Elements(numeric array=w1493) -> (sum=w1499:dbl)
                  n484 = Add Array Elements(numeric array=w1492) -> (sum=w1502:dbl)
                  n485 = Number To Fractional String(number=w1499) -> (F-format string=w1498:string)  [unwired: 3 in]
                  n486 = Number To Fractional String(number=w1502) -> (F-format string=w1500:string)  [unwired: 3 in]
                  n487 = Build Array (concatenate)(w1497, w1498, w1489, w1500, w1489, w1495, w1488, w1487) -> (w1501:string[])
                  n488 = Build Array (concatenate)(w1497, w1490) -> (w1496:string[])
                }
              }
            }
          }
        }
        n489 = Index Array(array=w1448) -> (element=w1449:string[])  [unwired: 2 in]
        n490 = for {
          tunnel: w1449 -> [_] mode=indexing
          tunnel: [w1457] -> w1447 mode=indexing
          i -> [w1458]
          n491 = Format Into String(w1458) -> (resulting string=w1457:string)  [unwired: 3 in, 1 out]
        }
        n492 = Replace Array Subset(array=w1447, new element="기기명" ("새 원소/부분배열"), index=0 ("인덱스")) -> (w1446:string[])
      }
    }
  }
  "에러 출력" <- w16
  "Data Out 2" <- w15
  "Data Out" <- w14
  "CalSTD" <- w13
